vi "EOL Save Module Test Data v2.6.vi"(8 "error in":errorcluster, 11 "main state cluster":T1={"Application Status"="", "Switch Output Array"=[], "Switch Value Configuration"=[], "NVH Configuration"={"NVH Station?"=FALSE, "nvh app instance path"="", "NVH_ErrorMessages sv url"="", "NVH_Inputs sv url"="", "NVH_MotionNumber sv url"="", "NVH_Outputs sv url"="", "NVH_PartNumber sv url"="", "NVH_PartNumber_Echo sv url"="", "NVH_SerialNumber sv url"="", "NVH_AmbientTempF sv url"=""}, "rs232 port map"={"PMAC"="", "PS Port"="", "LVDT Unit"="", "RS232"=""}, "ethernet address map"={"LVDT 1 Unit"="172.17.53.143", "LVDT Unit 1 port"=0}, "paths"={"Base Path"=path "", "system error log path"=path "", "Error Table Path"=path "C/Labview Code/System/Error Table", "Store errors log path"=path "C/Labview Code/System/Error Table", "data bytes log path"=path "C/Labview Code/System/Error Table", "network path"=path "C/Labview Code/System/Error Table"}, "Station Index"=0, "Store Data"={"Motion Data Array"=[], "Error Table"=[], "Sun Shade Close Force Limits"={"Overall Min"=0.0, "Overall Max"=0.0, "Avg Min"=0.0, "Avg Max"=0.0, "Truncation Start"=0.0, "Truncation End"=0.0, "Variance"=0.0, "Check Noise"=FALSE}, "Sun Shade Open Force Limits"={"Overall Min"=0.0, "Overall Max"=0.0, "Avg Min"=0.0, "Avg Max"=0.0, "Truncation Start"=0.0, "Truncation End"=0.0, "Variance"=0.0, "Check Noise"=FALSE}, "Sunshade Open Data"=[], "Sunshade Close Data"=[], "Module Info"={"Serial Number"="", "Pallet Number"="", "Sunshade Color"="", "Inalfa Part Number"="", "Customer Number"=""}, "Sunsahde Close Raw Data"=[], "Sunshade Open Raw Data"=[], "Software Version"=[], "Constant Version"=[], "Hardware Version"=[], "Inalfa Part Number ECU"=[], "LVDT Data"=[], "Communication Line 1"=[], "Communication Line 2"=[], "Anti Pinch Force"=[], "Cycle Time"="", "Anti Pinch Vent Force"=[], "iGPS LVDT Data"=[], "data bytes log"=""}, "D in map"={"Abort Test"=enum."Dev2/port2/line6", "Start Test"=enum."Dev2/port2/line6"}, "DO Task"="", "ctl refs"={"Start Test"=refnum, "Abort Test"=refnum, "Manual Control"=refnum, "Route to Repair"=refnum, "Waveform Graph"=refnum, "Motion Data"=refnum, "all station status"=refnum, "Individual Station Status"=refnum, "exit program"=refnum, "Sunshade Servo Data Open"=refnum, "Sunshade Servo Data Close"=refnum, "Red-Rabbit Mode"=refnum, "Direct Manual Ctrl"=refnum}, "misc station config"={"Station Name"="", "is AT station?"=FALSE, "is audit station?"=FALSE, "power supply type"=enum."GENser", "use alt China TP2 LVDT Logic Seq"=FALSE, "hmi operator abort timeout"=0, "dump all analog values even if pass"=FALSE, "debug log pre-filter ap stream bytes"=FALSE, "use separate lvdt x and z extend tags"=FALSE, "is print"=FALSE}, "ethernet tcp refs"={"LVDT Unit"=refnum}, "Sunshade Barcode Scan"={"Sunshade Number 2"="", "Sunshade Number 1"="", "Keyence tuning bank idx"=0}, "AP Test Data"={"Raw Sunshade AP Data"="", "Raw Glass AP Data"="", "PMAC Read Counter"=0.0, "Database AP Data"=[]}, "Motion Status"={"hmi operator abort start time"=0, "Current Data Index"=0, "Analog Data"=[], "Motor Position Hex"=0, "Messages Index"=0, "Last Bytes"=[], "Current Hall Position"=0, "Motion Stop Timer"=0, "Position Test"=enum."Not Tested", "Noise Test"=enum."Not Tested", "motion stop check initialized"=FALSE, "remote sense enabled"=FALSE, "Motion"=enum."Glass Teach"}, "LVDT Status"={"LVDT's stored config"=[], "lvdt precision"={"truncate instead of rounding"=FALSE, "decimal places"=0}}, "Sequence State"={"Step Description"="", "Cycle Start Time"=0, "Step Data String"="", "Pass?"=FALSE, "Seqence"=[], "Active Step"=0, "Testing?"=FALSE, "Red-Rabbit Mode"=FALSE, "route-to-repair mode"=FALSE, "NVH Status"={"Restart IRQ Counter"=0, "NVH Test Needed?"=FALSE, "NVH Test Running?"=FALSE}, "Present (s)"=0.0, "Hold Mode?"=FALSE, "Hold?"=FALSE, "Rx Invalid?"=FALSE}, "misc status"={"delay start time (ticks)"=0, "In Vehicle Mode?"=FALSE, "Diag Mode?"=FALSE, "Serial Port Configured?"=FALSE, "PS Voltage"=0.0, "Diag Serial Port"="", "Part Setup"={"Communication Type"=enum."None", "Send Messages to"=enum."Glass", "RAP Signal"=enum."High", "Motor Type"=enum."Smart Motor", "NVH Part Number"=0, "Turn Off Timer"=0, "Part Type"=""}, "Part History Number"="", "Plant Number"=0, "AP Data Type"=enum."91/61", "Real Rollo?"=FALSE}, "NVH Operator?"=FALSE, "NVH Pass?"=FALSE, "Operator Pass?"=FALSE, "Operator Action?"=FALSE, "Noise Source"=0, "USBHandle"=0, "PeakInfo"="", "PeakNumber"=0, "NVH Motion Steps"=[], "Second Check?"=FALSE, "Decibel data"=[], "Direct Control Info"={"EnableStopOnHome"=FALSE, "EnableStopOnPos"=FALSE, "TeachEvent"=FALSE, "open offset"=0, "close offset"=0, "Derect control"=FALSE, "set position"=[], "teach pass "=FALSE, "Drift offsets"=[], "Hall Positions"=[]}, "manual control(direct)"=FALSE, "LIN INFO"={"Toolkit Type"=enum."Inalfa LIN", "NAD"=36, "Inalfa LIN"={"Master Frame(3C)"="", "Slave Frame(3D)"="NIXNET_exampleLDF", "Request Schedule"="NIXNET_exampleLDF", "Response Schedule"="CEMLIN3DiagResponseSchedule\nSPA3414_ConfigurationsCMAGeely_CEMCALYPSOSDB34XX0Cfg_LIN3_190709_", "Frame Write SCU"="", "Frame Read SCU"="", "LIN Name"=""}, "ADCS LIN"={"Port"="MasterReq\nSPA3414_ConfigurationsCMAGeely_CEMCALYPSOSDB34XX0Cfg_LIN3_190709_", "HW select"=0, "XNET Cluster"="SlaveResp\nSPA3414_ConfigurationsCMAGeely_CEMCALYPSOSDB34XX0Cfg_LIN3_190709_", "ByteCmd Path"=path "C/Labview Code/System/ByteCmdConfig.txt"}, "TS LIN"={"ref info"=refnum, "LIN Channel"=0, "ByteCmd Path"=path "C/Labview Code/System/ByteCmdConfig.txt"}}, "Config Info"=variant} {"LIN INFO"."NAD" format="%.0x"; "LIN INFO"."ADCS LIN"."HW select" items=["NI-XNET", "NI-CAN"]; "LVDT Status"."LVDT's stored config"."Lower Limit" format="%.2f"; "LVDT Status"."LVDT's stored config"."Upper Limit" format="%.2f"; "Store Data"."Sun Shade Open Force Limits"."Variance" format="%.2g"; "Store Data"."Sun Shade Open Force Limits"."Truncation End" format="%.2g"; "Store Data"."Sun Shade Open Force Limits"."Truncation Start" format="%.2g"; "Store Data"."Sun Shade Open Force Limits"."Avg Max" format="%.2g"; "Store Data"."Sun Shade Open Force Limits"."Avg Min" format="%.2g"; "Store Data"."Sun Shade Open Force Limits"."Overall Max" format="%.2g"; "Store Data"."Sun Shade Open Force Limits"."Overall Min" format="%.2g"; "Store Data"."Sun Shade Close Force Limits"."Variance" format="%.2g"; "Store Data"."Sun Shade Close Force Limits"."Truncation End" format="%.2g"; "Store Data"."Sun Shade Close Force Limits"."Truncation Start" format="%.2g"; "Store Data"."Sun Shade Close Force Limits"."Avg Max" format="%.2g"; "Store Data"."Sun Shade Close Force Limits"."Avg Min" format="%.2g"; "Store Data"."Sun Shade Close Force Limits"."Overall Max" format="%.2g"; "Store Data"."Sun Shade Close Force Limits"."Overall Min" format="%.2g"; "Store Data"."Motion Data Array"."Motion Data Limits"."LIN Msg"."Msg" format="%02x"; "Store Data"."Motion Data Array"."Motion Data Limits"."LIN Msg"."ID" format="%02x"}) -> (0 "error out":errorcluster)   [LabVIEW 2018]
uses:
  02.Type Def's/main state cluster.ctl
  02.Type Def's/All Switch Configuration Cluster.ctl
  02.Type Def's/All Motions.ctl
  02.Type Def's/EOL Switch Value Configuration Cluster.ctl
  02.Type Def's/EOL Switch Max Min Check Cluster.ctl
  02.Type Def's/station nvh config.ctl
  02.Type Def's/station rs232 port map.ctl
  02.Type Def's/station ethernet address map.ctl
  02.Type Def's/station paths.ctl
  02.Type Def's/EOL Save Module Test Data Control.ctl
  02.Type Def's/EOL Motion Database Table.ctl
  05.UserVI's/type defs/17x Audit Motion Data Seq Control.ctl
  05.UserVI's/type defs/17x AP Data Type.ctl
  05.UserVI's/type defs/17x Sunshade Limts Seq.ctl
  02.Type Def's/EOL Module Info Control.ctl
  02.Type Def's/station DI map.ctl
  05.UserVI's/type defs/EOL Global Digital Input Control.ctl
  02.Type Def's/control refs.ctl
  02.Type Def's/station motion data indicator.ctl
  02.Type Def's/Screen Motion Data.ctl
  02.Type Def's/Pass Fail Control.ctl
  02.Type Def's/station hmi.ctl
  02.Type Def's/lvdt name val pair.ctl
  02.Type Def's/individual station status.ctl
  02.Type Def's/misc station config.ctl
  05.UserVI's/Lambda Power/power supply types.ctl
  05.UserVI's/type defs/EOL LVDT's Check Controller.ctl
  05.UserVI's/LVDT's/lvdt precision.ctl
  02.Type Def's/sequence state.ctl
  05.UserVI's/sequence/type defs/Sequence Info.ctl
  05.UserVI's/type defs/EOL Part Setup.ctl
  02.Type Def's/All Communication Types.ctl
  05.UserVI's/type defs/Communication with Motors.ctl
  05.UserVI's/type defs/RAP Signal Control.ctl
  05.UserVI's/type defs/EOL Motor Type.ctl
  02.Type Def's/station LIN config.ctl
  03.Inalfa LIN/LIN Device.ctl
  <vilib>/CMC.AME/Inalfa ADCS/Ctl'Def/ADCS_LIN info.ctl
  C:/Program Files (x86)/National Instruments/LabVIEW 2018/vi.lib/CMC.AME/Inalfa TS LIN/TOSUN/TSMaster/bin/Interop.TSMasterAPI.dll
  Program Files (x86)/National Instruments/LabVIEW 2018/vi.lib/CMC.AME/Inalfa TS LIN/TOSUN/TSMaster/bin/Interop.TSMasterAPI.dll
  06.Test Loop/Sub'VIs/Type Def's/Config Info.ctl
  <vilib>/Utility/file.llb/Write To Spreadsheet File (string).vi
panel:
  in  "Store Sunshade Raw Data?":bool
  # "Sunroof Barcode"
  # "Pallet Number"
  # "Part Type"
  # "Application Status"
  # "Current Step"
  # "Cycle Time"
  # "Pass / Fail"
  # "Shade Close"
  # "Actual Data"
  # "Limits"
  # "Avg Current"
  # "Run Time"
  # "Speed"
  # "Noise Test"
  # "Position"
  # "Shade Open"
  # "Actual Data"
  # "Limits"
  # "Avg Current"
  # "Run Time"
  # "Speed"
  # "Noise Test"
  # "Position"
  # "Vent Close"
  # "Actual Data"
  # "Limits"
  # "Avg Current"
  # "Run Time"
  # "Speed"
  # "Noise Test"
  # "Position"
  # "Vent Open"
  # "Actual Data"
  # "Limits"
  # "Avg Current"
  # "Run Time"
  # "Speed"
  # "Noise Test"
  # "Position"
  # "Slide Close"
  # "Actual Data"
  # "Limits"
  # "Avg Current"
  # "Run Time"
  # "Speed"
  # "Noise Test"
  # "Position"
  # "Slide Open"
  # "Actual Data"
  # "Limits"
  # "Avg Current"
  # "Run Time"
  # "Speed"
  # "Noise Test"
  # "Position"
  # "Min"
  # "N"
  # "Min"
  # "Start"
  # "N"
  # "Max"
  # "N"
  # "Max"
  # "N"
  # "End"
  # "Min"
  # "N"
  # "Min"
  # "Start"
  # "N"
  # "Max"
  # "N"
  # "Max"
  # "N"
  # "End"
  # "Min"
  # "Max"
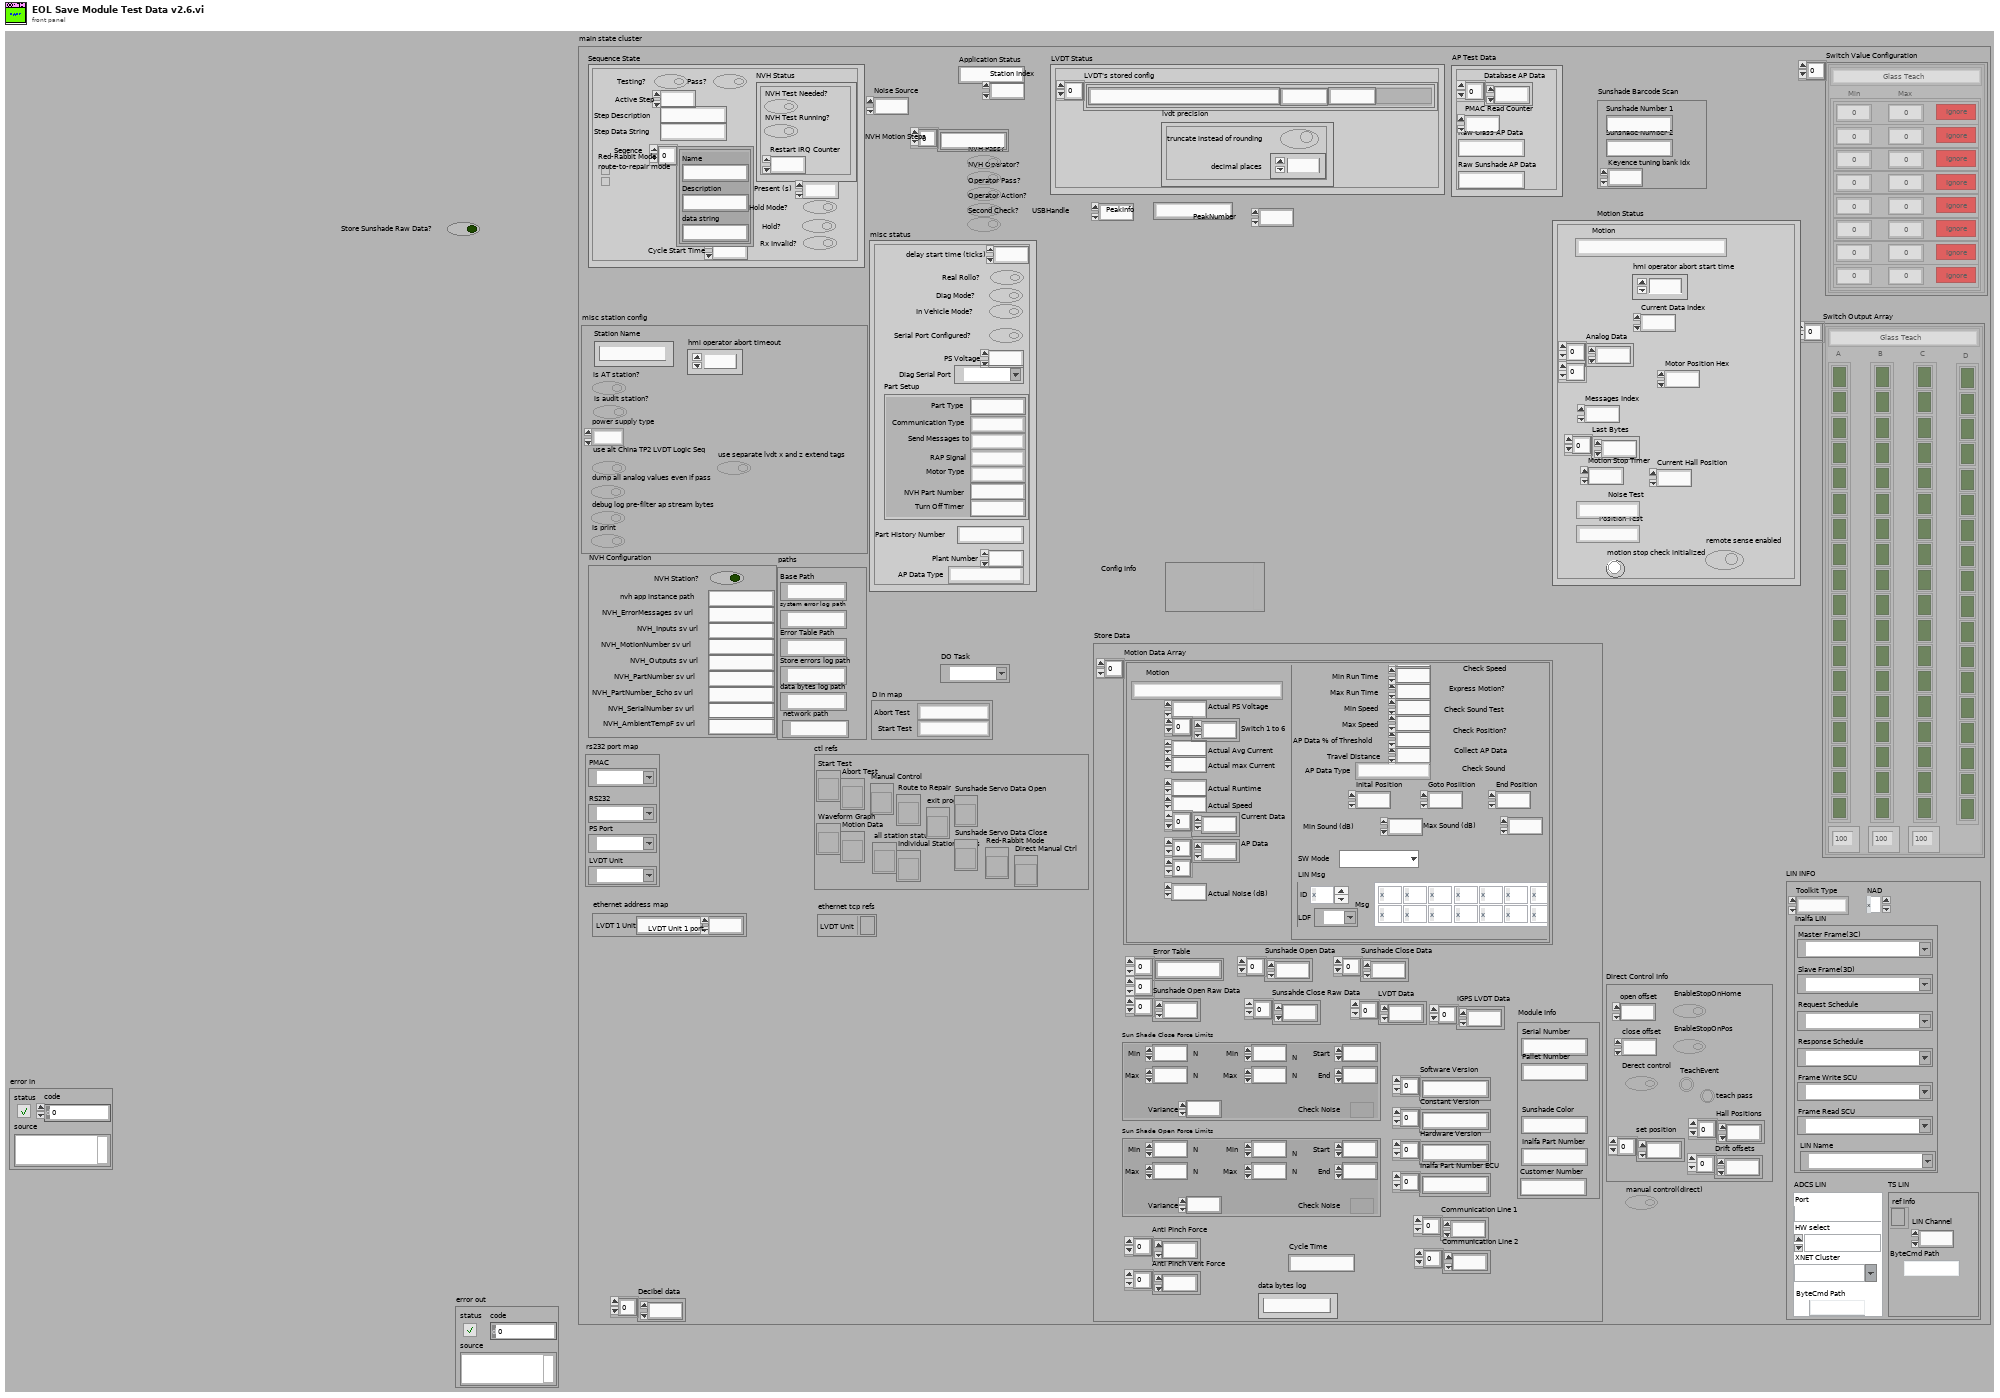
[diagram p1: front panel]
types:
  T1 = typedef "main state cluster.ctl" = cluster{"Application Status":string, "Switch Output Array":T2[], "Switch Value Configuration":T4[], "NVH Configuration":T6, "rs232 port map":T7, "ethernet address map":T8, "paths":T9, "Station Index":i32, "Store Data":T10, "D in map":T16, "DO Task":refnum<k21>, "ctl refs":T18, "misc station config":T19, "ethernet tcp refs":cluster{"LVDT Unit":refnum<k5>}, "Sunshade Barcode Scan":cluster{"Sunshade Number 2":string, "Sunshade Number 1":string, "Keyence tuning bank idx":i32}, "AP Test Data":cluster{"Raw Sunshade AP Data":string, "Raw Glass AP Data":string, "PMAC Read Counter":dbl, "Database AP Data":dbl[]}, "Motion Status":cluster{"hmi operator abort start time":u32, "Current Data Index":i32, "Analog Data":sgl[][], "Motor Position Hex":u16, "Messages Index":u16, "Last Bytes":u8[], "Current Hall Position":i16, "Motion Stop Timer":u32, "Position Test":T21, "Noise Test":T21, "motion stop check initialized":bool, "remote sense enabled":bool, "Motion":T3}, "LVDT Status":cluster{"LVDT's stored config":T22[], "lvdt precision":T23}, "Sequence State":T24, "misc status":cluster{"delay start time (ticks)":u32, "In Vehicle Mode?":bool, "Diag Mode?":bool, "Serial Port Configured?":bool, "PS Voltage":dbl, "Diag Serial Port":refnum<visa-resource-name>, "Part Setup":T26, "Part History Number":string, "Plant Number":u8, "AP Data Type":T13, "Real Rollo?":bool}, "NVH Operator?":bool, "NVH Pass?":bool, "Operator Pass?":bool, "Operator Action?":bool, "Noise Source":u32, "USBHandle":i32, "PeakInfo":string, "PeakNumber":i32, "NVH Motion Steps":string[], "Second Check?":bool, "Decibel data":dbl[], "Direct Control Info":cluster{"EnableStopOnHome":bool, "EnableStopOnPos":bool, "TeachEvent":bool, "open offset":i32, "close offset":i32, "Derect control":bool, "set position":i32[], "teach pass ":bool, "Drift offsets":i32[], "Hall Positions":i32[]}, "manual control(direct)":bool, "LIN INFO":T31, "Config Info":T34}
  T2 = typedef "All Switch Configuration Cluster.ctl" = cluster{"All Motions":T3, "A":bool[], "B":bool[], "C":bool[], "D":bool[], "A activation time (ms)":u32, "B activation time (ms)":u32, "C activation time (ms)":u32}
  T3 = typedef "All Motions.ctl" = enum16{"Glass Teach", "Glass Slide Open", "Glass Slide Close", "Glass Vent Open", "Glass Vent Close", "Sunshade Teach", "Sunshade Open", "Sunshade Close", "Idle", "Sunshade Open 2", "Sunshade Close 2", "Glass Slide Open Sunshade Open", "Glass Slide Open Sunshade Close", "Glass Slide Close Sunshade Open", "Glass Slide Close Sunshade Close", "Glass Vent Open Sunshade Open", "Glass Vent Open Sunshade Close", "Glass Vent Close Sunshade Open", "Glass Vent Close Sunshade Close", "Express Glass Slide Open", "Express Glass Slide Close", "Express Glass Vent Open", "Express Glass Vent Close", "Express Sunshade Open", "Express Sunshade Close", "Express Sunshade Open 2", "Express Sunshade Close 2", "Express Glass Slide Open Sunshade Open", "Express Glass Slide Open Sunshade Close", "Express Glass Slide Close Sunshade Open", "Express Glass Slide Close Sunshade Close", "Express Glass Vent Open Sunshade Open", "Express Glass Vent Open Sunshade Close", "Express Glass Vent Close Sunshade Open", "Express Glass Vent Close Sunshade Close", "Goto Position Glass", "Goto Position Sunshade", "Sunshade Teach 2"}
  T4 = typedef "EOL Switch Value Configuration Cluster.ctl" = cluster{"All Motions":T3, "Array":T5[]}
  T5 = typedef "EOL Switch Max Min Check Cluster.ctl" = cluster{"Min":dbl, "Max":dbl, "Check?":bool}
  T6 = typedef "station nvh config.ctl" = cluster{"NVH Station?":bool, "nvh app instance path":string, "NVH_ErrorMessages sv url":string, "NVH_Inputs sv url":string, "NVH_MotionNumber sv url":string, "NVH_Outputs sv url":string, "NVH_PartNumber sv url":string, "NVH_PartNumber_Echo sv url":string, "NVH_SerialNumber sv url":string, "NVH_AmbientTempF sv url":string}
  T7 = typedef "station rs232 port map.ctl" = cluster{"PMAC":refnum<visa-resource-name>, "PS Port":refnum<visa-resource-name>, "LVDT Unit":refnum<visa-resource-name>, "RS232":refnum<visa-resource-name>}
  T8 = typedef "station ethernet address map.ctl" = cluster{"LVDT 1 Unit":string, "LVDT Unit 1 port":u16}
  T9 = typedef "station paths.ctl" = cluster{"Base Path":path, "system error log path":path, "Error Table Path":path, "Store errors log path":path, "data bytes log path":path, "network path":path}
  T10 = typedef "EOL Save Module Test Data Control.ctl" = cluster{"Motion Data Array":T11[], "Error Table":string[][], "Sun Shade Close Force Limits":T14, "Sun Shade Open Force Limits":T14, "Sunshade Open Data":sgl[], "Sunshade Close Data":sgl[], "Module Info":T15, "Sunsahde Close Raw Data":sgl[], "Sunshade Open Raw Data":sgl[], "Software Version":string[], "Constant Version":string[], "Hardware Version":string[], "Inalfa Part Number ECU":string[], "LVDT Data":sgl[], "Communication Line 1":sgl[], "Communication Line 2":sgl[], "Anti Pinch Force":sgl[], "Cycle Time":string, "Anti Pinch Vent Force":sgl[], "iGPS LVDT Data":sgl[], "data bytes log":string}
  T11 = typedef "EOL Motion Database Table.ctl" = cluster{"Motion":T3, "Actual Avg Current":dbl, "Actual Runtime":dbl, "Actual Speed":dbl, "Current Data":sgl[], "Motion Data Limits":T12, "Switch 1 to 6":dbl[], "Actual PS Voltage":dbl, "AP Data":i16[][], "Actual max Current":dbl, "Actual Noise (dB)":dbl}
  T12 = typedef "17x Audit Motion Data Seq Control.ctl" = cluster{"Power Supply Voltage":dbl, "Min Avg Current":dbl, "Max Avg Current":dbl, "Min Run Time":dbl, "Max Run Time":dbl, "Min Speed":dbl, "Max Speed":dbl, "AP Data % of Threshold":dbl, "Travel Distance":dbl, "AP Data Type":T13, "Check Current":bool, "Check Run Time":bool, "Check Speed":bool, "Express Motion?":bool, "Check Sound Test":bool, "Check Position?":bool, "Collect AP Data":bool, "Inital Position":u16, "End Position":u16, "Goto Posiition":u16, "Max max Current":dbl, "Min max Current":dbl, "Check max Current":bool, "Check Sound":bool, "Min Sound (dB)":dbl, "Max Sound (dB)":dbl, "SW Mode":enum16{"Hard Switch", "Uncond Frame"}, "LIN Msg":cluster{"ID":u8, "Msg":u8[][], "LDF":refnum<k21>}}
  T13 = typedef "17x AP Data Type.ctl" = enum16{"91/61", "92/62", "93/63", "67", "68", "6F", "71", "91 Msg", "92 Msg", "93 Msg", "94 Msg", "HiRain 91", "HiRain 92 Speed", "HiRain 92 HS", "HiRain 92", "HiRain 93", "SnT"}
  T14 = typedef "17x Sunshade Limts Seq.ctl" = cluster{"Overall Min":dbl, "Overall Max":dbl, "Avg Min":dbl, "Avg Max":dbl, "Truncation Start":dbl, "Truncation End":dbl, "Variance":dbl, "Check Noise":bool}
  T15 = typedef "EOL Module Info Control.ctl" = cluster{"Serial Number":string, "Pallet Number":string, "Sunshade Color":string, "Inalfa Part Number":string, "Customer Number":string}
  T16 = typedef "station DI map.ctl" = cluster{"Abort Test":T17, "Start Test":T17}
  T17 = typedef "EOL Global Digital Input Control.ctl" = enum16{"Dev2/port0/line0", "Dev2/port0/line1", "Dev2/port0/line2", "Dev2/port0/line3", "Dev2/port0/line4", "Dev2/port0/line5", "Dev2/port0/line6", "Dev2/port0/line7", "Dev2/port1/line0", "Dev2/port1/line1", "Dev2/port1/line2", "Dev2/port1/line3", "Dev2/port1/line4", "Dev2/port1/line5", "Dev2/port1/line6", "Dev2/port1/line7", "Dev2/port2/line0", "Dev2/port2/line1", "Dev2/port2/line2", "Dev2/port2/line3", "Dev2/port2/line4", "Dev2/port2/line5", "Dev2/port2/line6", "Dev2/port2/line7", "Prerun Start Test", "Prerun Abort Test", "Audit Start Test", "Audit Abort Test", "Dev2/port3/line4", "Dev2/port3/line5", "Breakin Start Test", "Breakin Abort Test", "Not Implemented"}
  T18 = typedef "control refs.ctl" = cluster{"Start Test":refnum<vi>, "Abort Test":refnum<vi>, "Manual Control":refnum<vi>, "Route to Repair":refnum<vi>, "Waveform Graph":refnum<vi>, "Motion Data":refnum<vi>, "all station status":refnum<vi>, "Individual Station Status":refnum<vi>, "exit program":refnum<vi>, "Sunshade Servo Data Open":refnum<vi>, "Sunshade Servo Data Close":refnum<vi>, "Red-Rabbit Mode":refnum<vi>, "Direct Manual Ctrl":refnum<vi>}
  T19 = typedef "misc station config.ctl" = cluster{"Station Name":string, "is AT station?":bool, "is audit station?":bool, "power supply type":T20, "use alt China TP2 LVDT Logic Seq":bool, "hmi operator abort timeout":u32, "dump all analog values even if pass":bool, "debug log pre-filter ap stream bytes":bool, "use separate lvdt x and z extend tags":bool, "is print":bool}
  T20 = typedef "power supply types.ctl" = enum16{"GENser", "ZUPser", "GENeth", "Manual", "ITECH"}
  T21 = typedef "Pass Fail Control.ctl" = enum16{"Not Tested", "Pass", "Fail"}
  T22 = typedef "EOL LVDT's Check Controller.ctl" = cluster{"Upper Limit":dbl, "Lower Limit":dbl, "LVDT Name":string, "Check":bool}
  T23 = typedef "lvdt precision.ctl" = cluster{"truncate instead of rounding":bool, "decimal places":u8}
  T24 = typedef "sequence state.ctl" = cluster{"Step Description":string, "Cycle Start Time":u32, "Step Data String":string, "Pass?":bool, "Seqence":T25[], "Active Step":u8, "Testing?":bool, "Red-Rabbit Mode":bool, "route-to-repair mode":bool, "NVH Status":cluster{"Restart IRQ Counter":u8, "NVH Test Needed?":bool, "NVH Test Running?":bool}, "Present (s)":dbl, "Hold Mode?":bool, "Hold?":bool, "Rx Invalid?":bool}
  T25 = typedef "Sequence Info.ctl" = cluster{"Name":string, "Description":string, "data string":string}
  T26 = typedef "EOL Part Setup.ctl" = cluster{"Communication Type":T27, "Send Messages to":T28, "RAP Signal":T29, "Motor Type":T30, "NVH Part Number":u16, "Turn Off Timer":u16, "Part Type":string}
  T27 = typedef "All Communication Types.ctl" = enum16{"None", "CAN", "RS 232", "RS 232 LIN", "GM LIN", "SnT LIN", "K Line", "Robel CAN", "P42M-Continental", "Inalfa SCU LIN", "Spare 3"}
  T28 = typedef "Communication with Motors.ctl" = enum16{"Glass", "Rollo", "Both"}
  T29 = typedef "RAP Signal Control.ctl" = enum16{"High", "Low", "None"}
  T30 = typedef "EOL Motor Type.ctl" = enum16{"Smart Motor", "Sensor Motor"}
  T31 = typedef "station LIN config.ctl" = cluster{"Toolkit Type":enum16{"Inalfa LIN", "ADCS LIN", "TS LIN"}, "NAD":u8, "Inalfa LIN":T32, "ADCS LIN":T33, "TS LIN":cluster{"ref info":refnum<k24>, "LIN Channel":i32, "ByteCmd Path":path}}
  T32 = typedef "LIN Device.ctl" = cluster{"Master Frame(3C)":refnum<k21>, "Slave Frame(3D)":refnum<k21>, "Request Schedule":refnum<k21>, "Response Schedule":refnum<k21>, "Frame Write SCU":refnum<k21>, "Frame Read SCU":refnum<k21>, "LIN Name":refnum<k21>}
  T33 = typedef "ADCS_LIN info.ctl" = cluster{"Port":string, "HW select":u16, "XNET Cluster":string, "ByteCmd Path":path}
  T34 = typedef "Config Info.ctl" = variant
  T35 = cluster{"Base Path":path, "Relative Path Excel Data":string, "Relative Path AP Data":string, "Relative Path Current Data":string, "Relative Path Sunshade Force Data":string, "Excel Data Array":string[], "Date n Time":string, "AP Data":i16[][][], "Current Data":sgl[][], "Relative Path Data Bytes Log":string, "Relative Path Analog Data":string, "main state cluster":T1, "Red Rabbit Relative Path Excel Data":string, "Route to repair relative path excel data":string, "bmw hall log relative path":string}
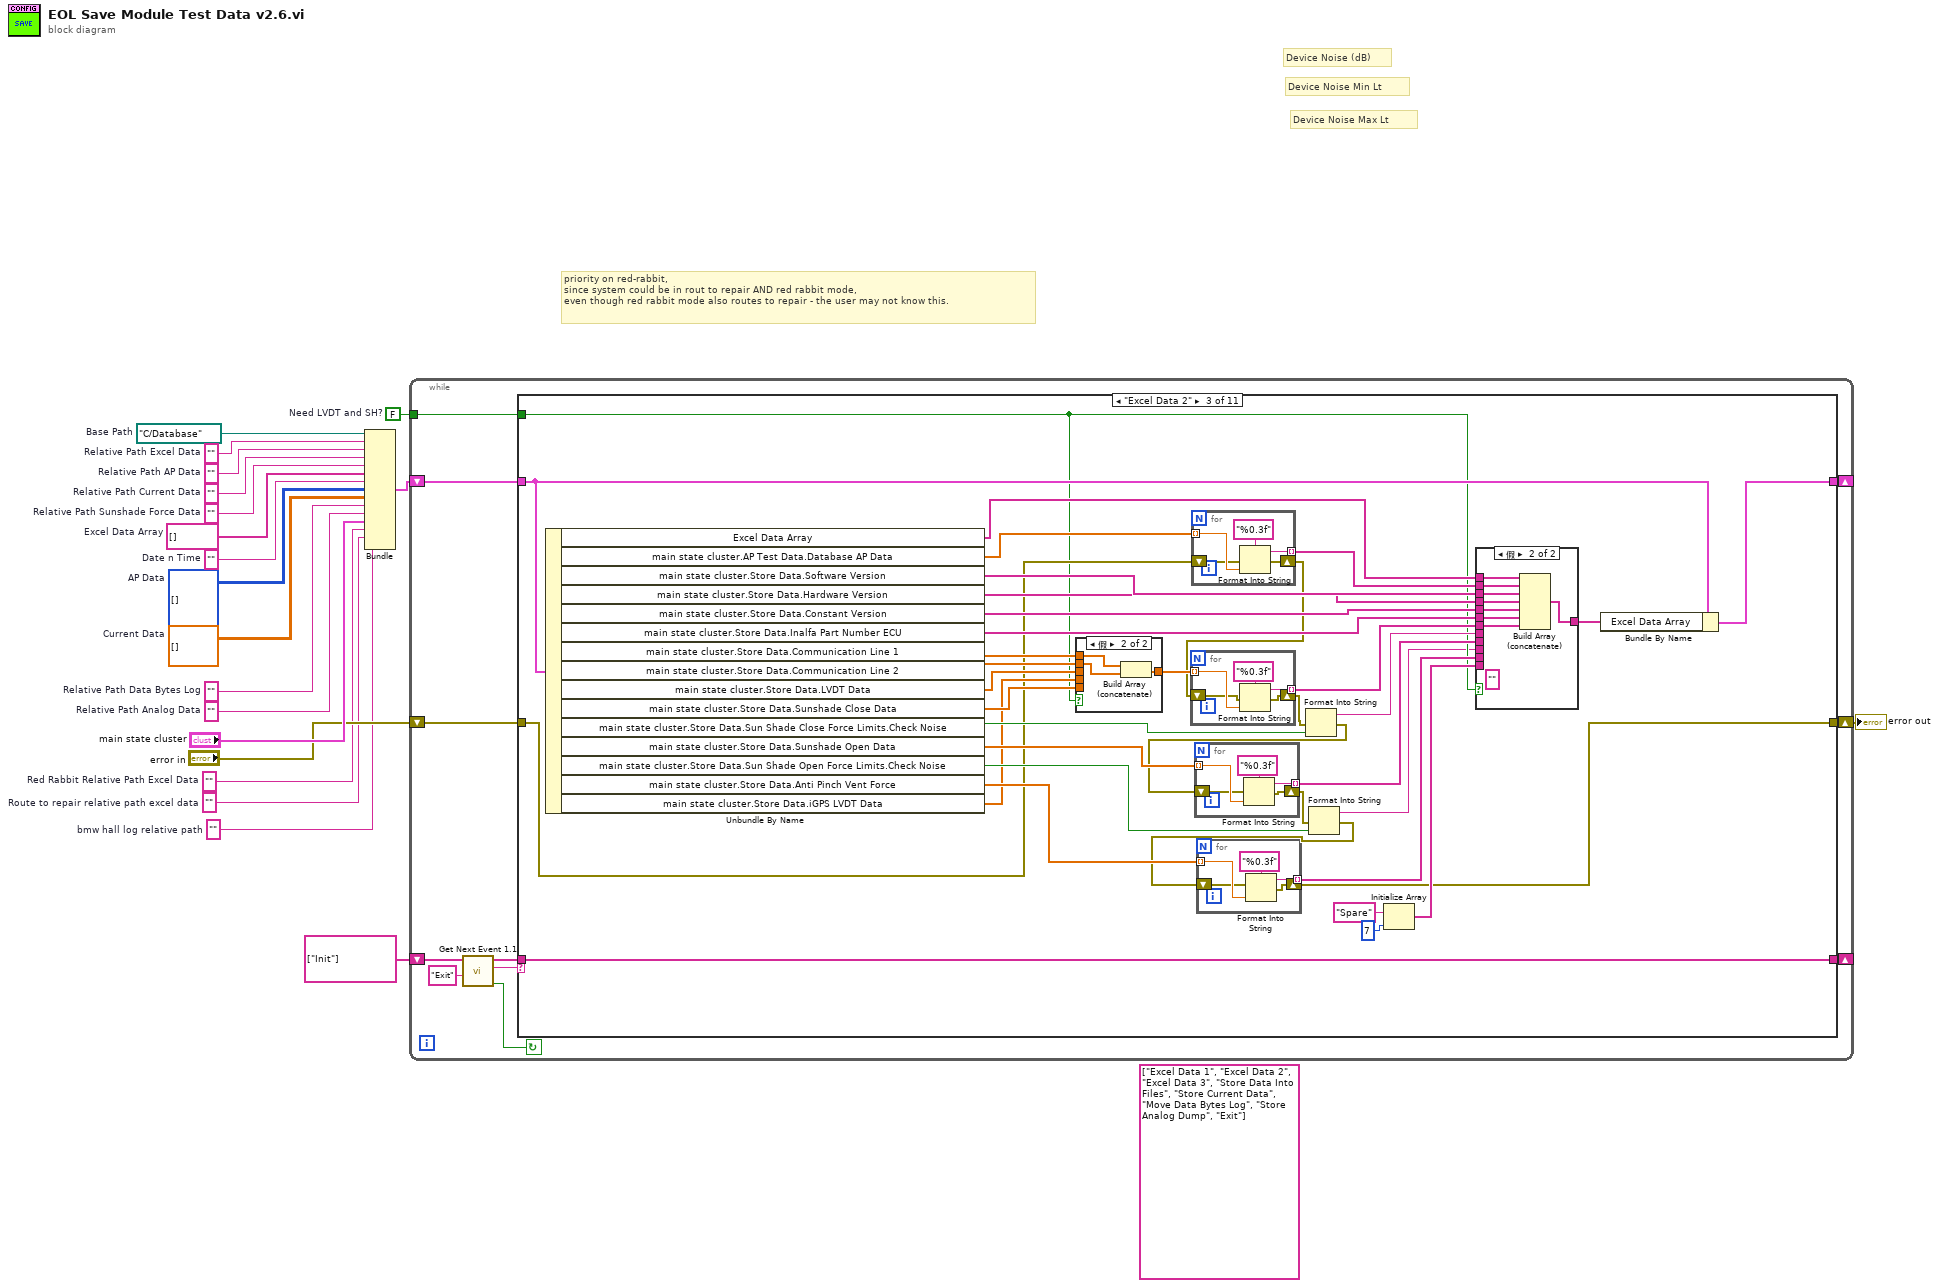
[diagram p0: block diagram]
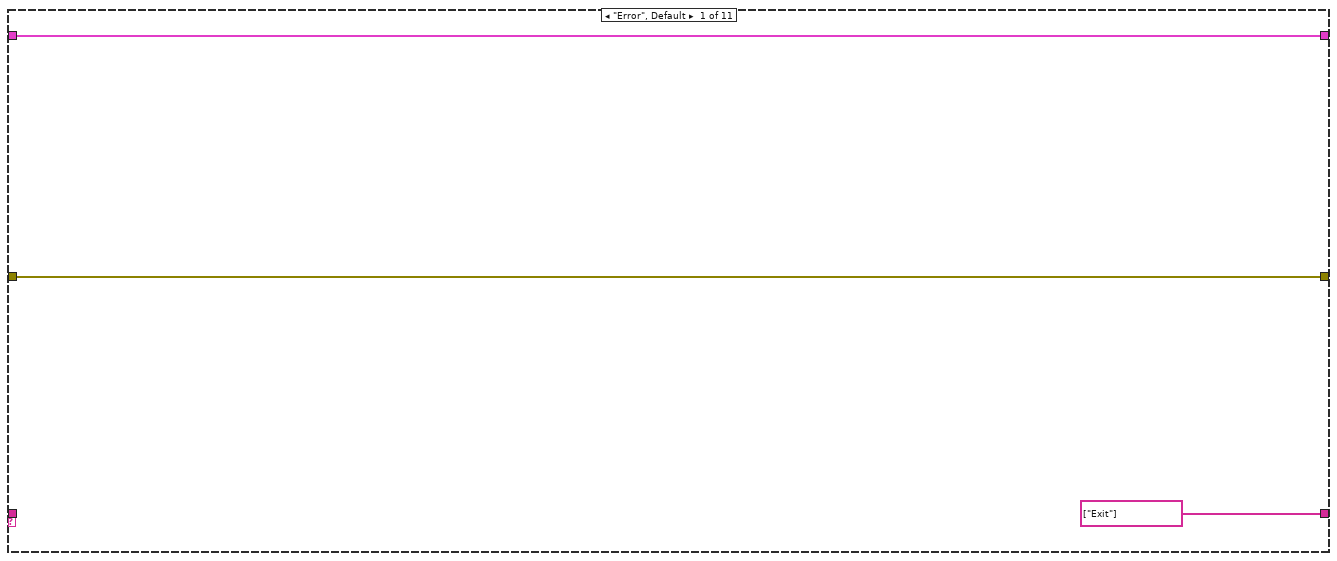
[diagram p2: hidden frame]
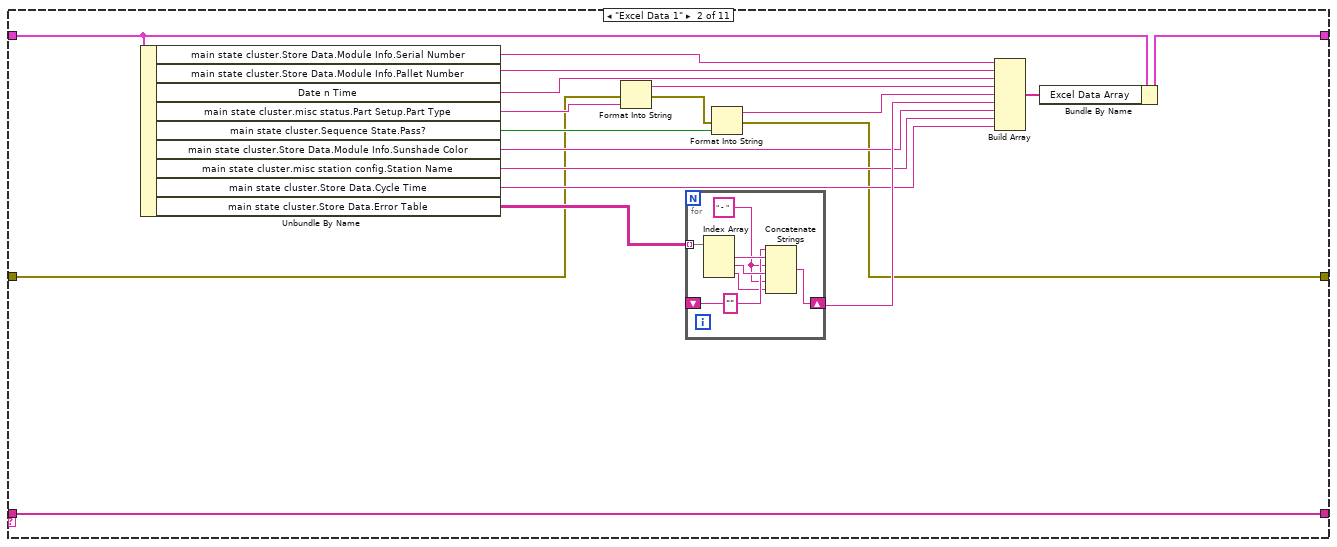
[diagram p3: hidden frame]
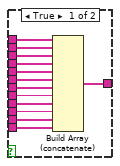
[diagram p4: hidden frame]
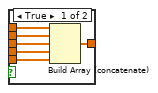
[diagram p5: hidden frame]
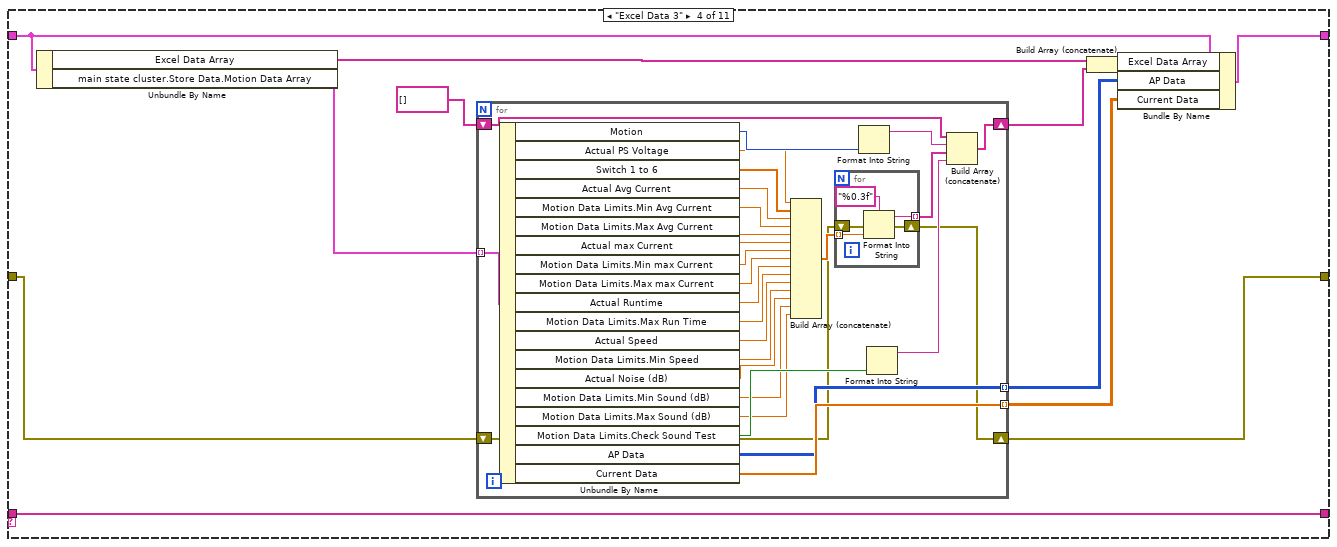
[diagram p6: hidden frame]
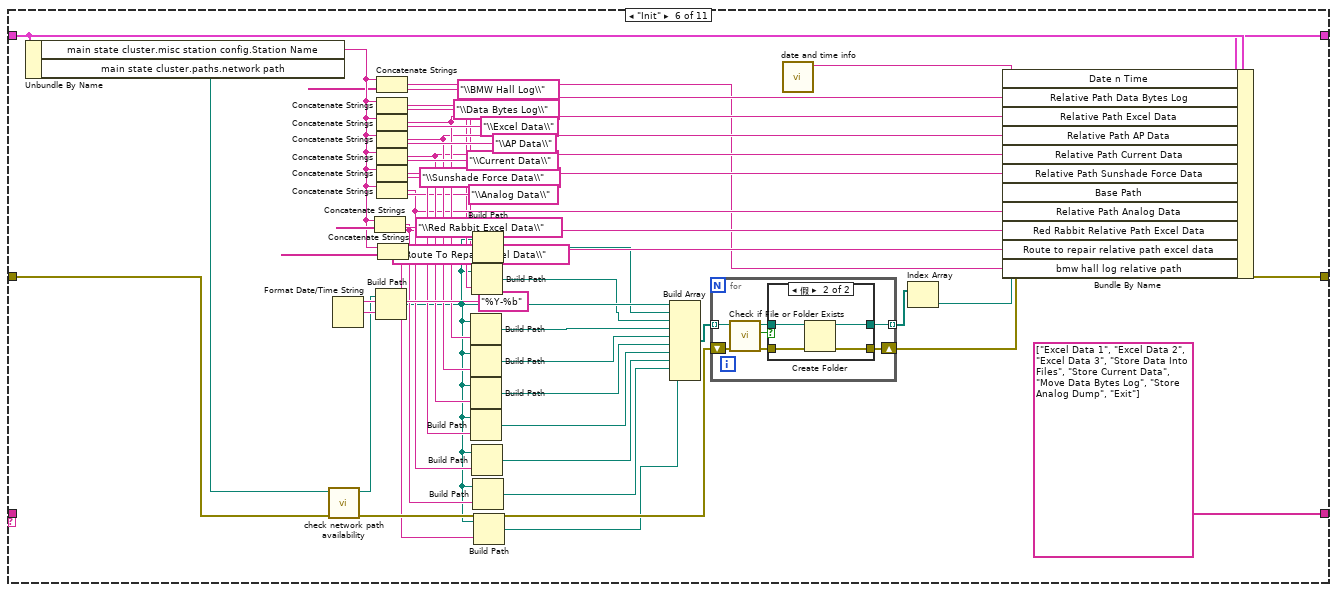
[diagram p8: hidden frame]
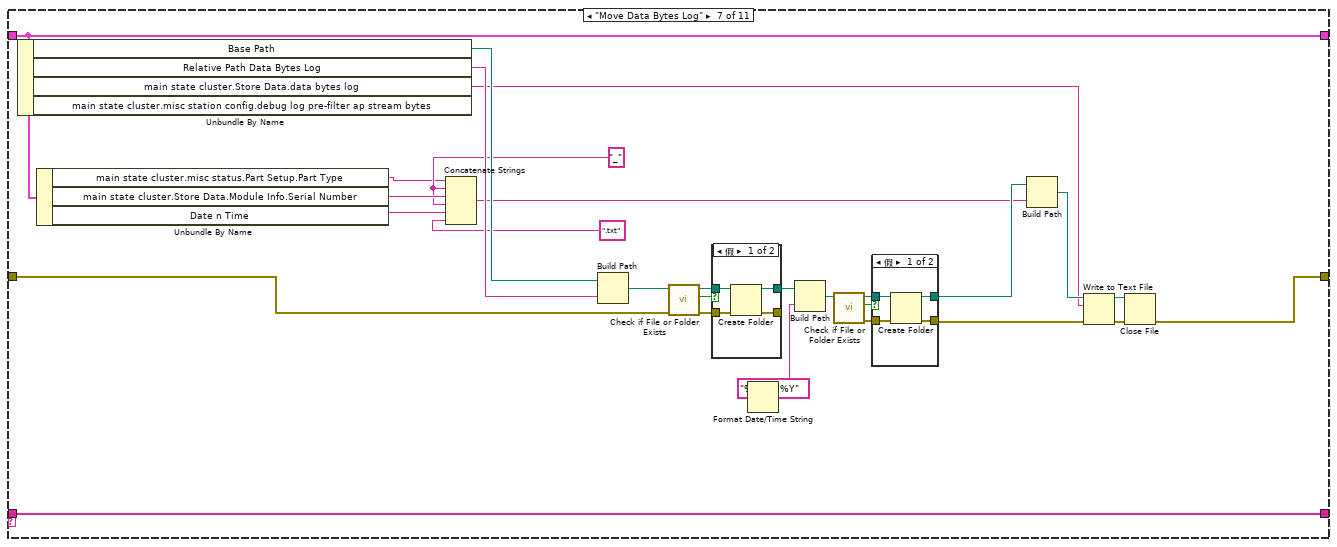
[diagram p10: hidden frame]
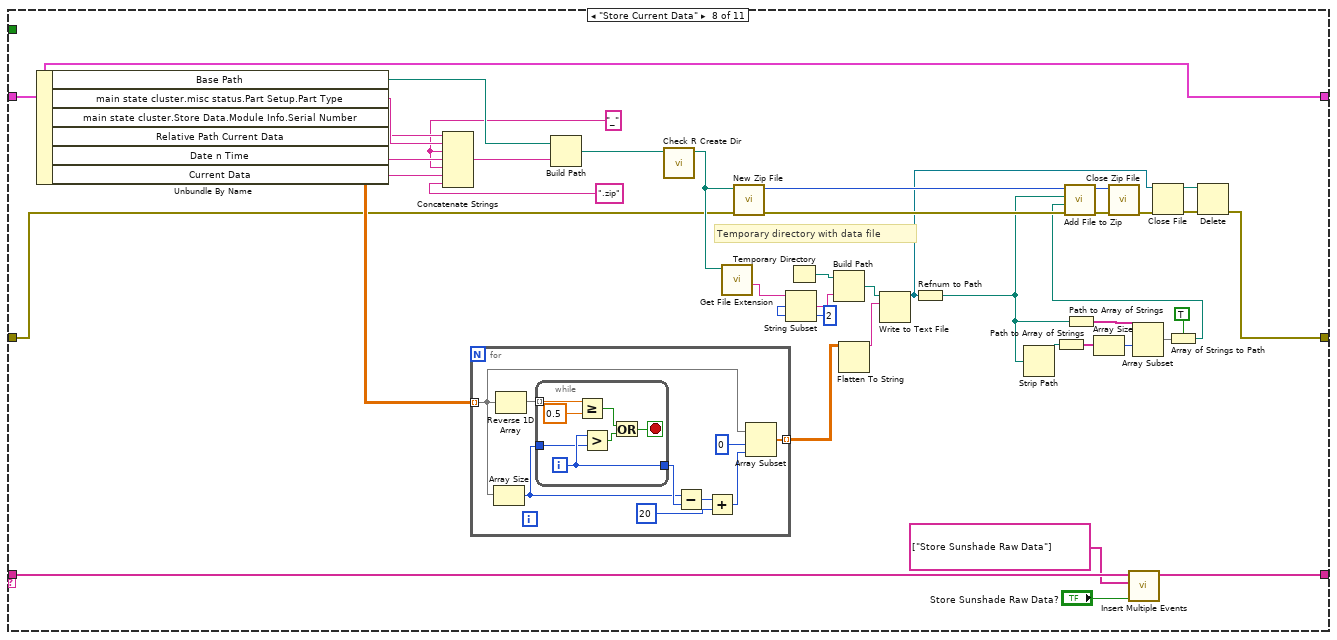
[diagram p13: hidden frame]
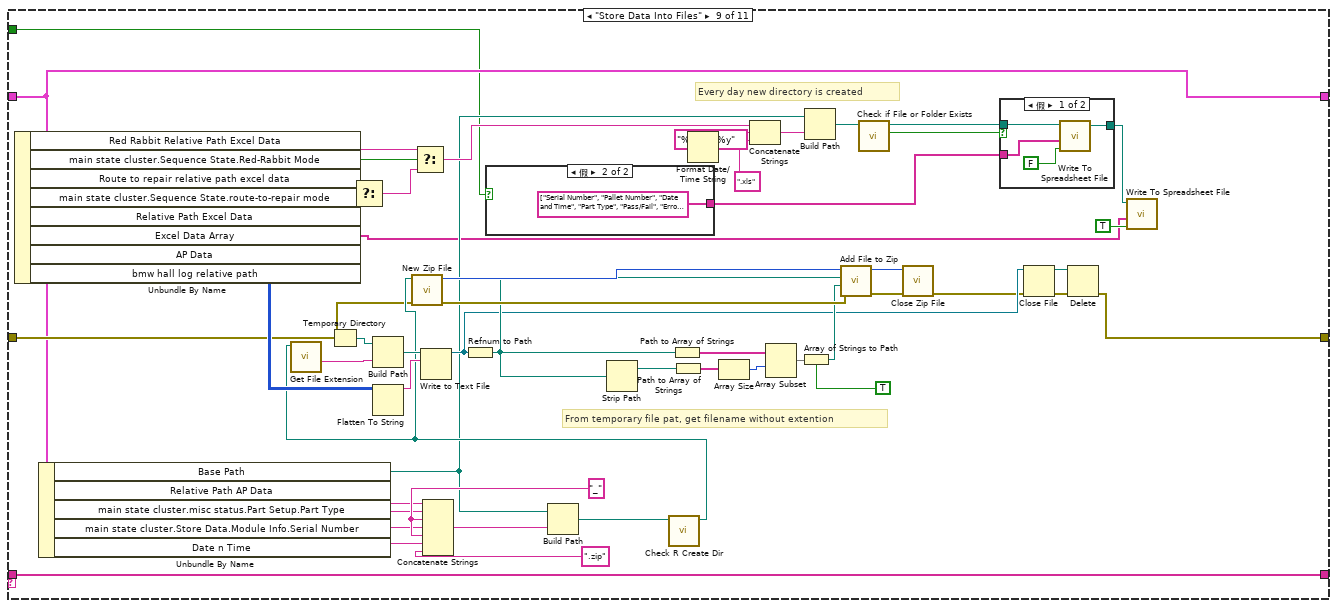
[diagram p14: hidden frame]
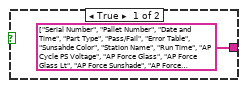
[diagram p15: hidden frame]
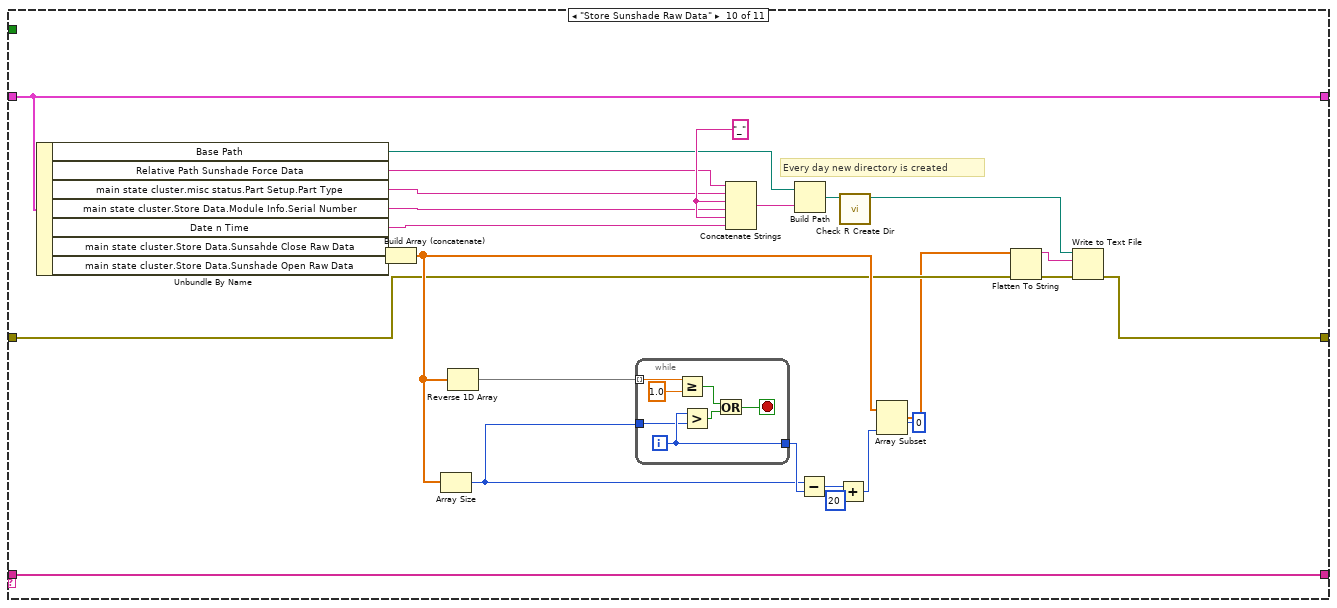
[diagram p17: hidden frame]
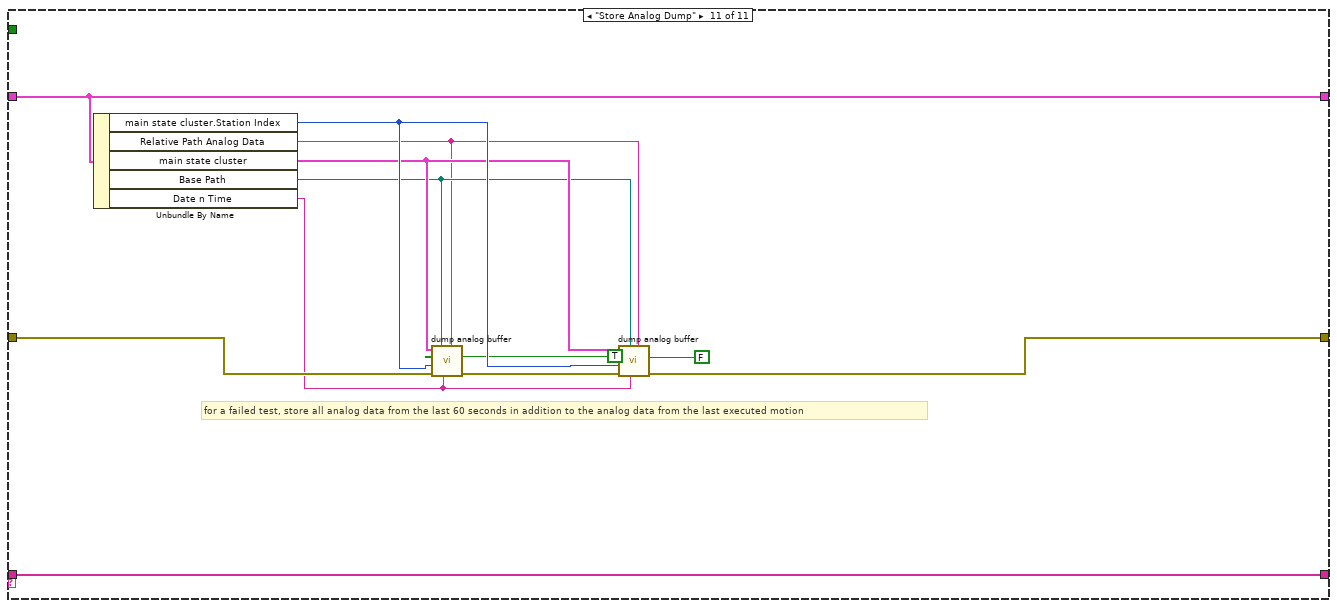
[diagram p18: hidden frame]
diagram:
  w1 = FALSE  # Need LVDT and SH?
  (unwired) string[] ["Excel Data 1", "Excel Data 2", "Excel Data 3", "Store Data Into Files", "Store Current Data", "Move Data Bytes Log", "Store Analog Dump", "Exit"] ("event queue out")
  w2 = ""  # bmw hall log relative path
  w3 = ""  # Route to repair relative path excel data
  w4 = ""  # Red Rabbit Relative Path Excel Data
  w8 = ""  # Relative Path Analog Data
  w9 = ""  # Relative Path Data Bytes Log
  w19 = path "C:/Database"  # Base Path
  w10 = sgl[][] []  # Current Data
  w11 = i16[][][] []  # AP Data
  w12 = ""  # Date n Time
  w13 = string[] []  # Excel Data Array
  w14 = ""  # Relative Path Sunshade Force Data
  w15 = ""  # Relative Path Current Data
  w16 = ""  # Relative Path AP Data
  w17 = ""  # Relative Path Excel Data
  # "priority on red-rabbit,\nsince system could be in rout to repair AND red rabbit mode,\neven though red rabbit mode also routes to repair - the user may not know this."
  # "Device Noise Max Lt"
  # "Device Noise Min Lt"
  # "Device Noise (dB)"
  n1 = Bundle("Base Path"=w19, "Relative Path Excel Data"=w17, "Relative Path AP Data"=w16, "Relative Path Current Data"=w15, "Relative Path Sunshade Force Data"=w14, "Excel Data Array"=w13, "Date n Time"=w12, "AP Data"=w11, "Current Data"=w10, "Relative Path Data Bytes Log"=w9, "Relative Path Analog Data"=w8, "main state cluster"="main state cluster", "Red Rabbit Relative Path Excel Data"=w4, "Route to repair relative path excel data"=w3, "bmw hall log relative path"=w2) -> (w18:T35)  [unwired: 1 in]
  n2 = while {
    shift-right: [w28] -> _
    shift-left: string[] ["Init"] ("event queue out") -> [w27]
    shift-right: [w25] -> _
    shift-left: w18 -> [w26]
    shift-right: [w22] -> w5
    shift-left: "error in" -> [w23]
    tunnel: w1 -> [w21]
    stop <- w31 continue-if-true
    n3 = call "Get Next Event 1.1.vi"("Exit Event"="Exit", "event queue in"=w27) -> ("Condition (Exit:F)"=w31:bool, "next event"=w30:string, "event queue out"=w29:string[])  [unwired: 6 in, 1 out]
    n4 = case shown="\"Excel Data 2\"" w30 {
      tunnel: w29 -> [_ w54 w98 w160 w195 _ w275 w333 w390 w437 w453]
      tunnel: [string[] ["Exit"] ("event queue out") w54 w98 w160 w195 string[] ["Excel Data 1", "Excel Data 2", "Excel Data 3", "Store Data Into Files", "Store Current Data", "Move Data Bytes Log", "Store Analog Dump", "Exit"] ("event queue out") w275 w332 w390 w437 w453] -> w28
      tunnel: w26 -> [w34 w51 w96 w159 w196 w239 w261 w296 w354 w413 w454]
      tunnel: [w34 w50 w95 w158 w196 w238 w261 w296 w354 w413 w454] -> w25
      tunnel: w23 -> [w32 w37 w70 w150 w194 w213 w266 w294 w364 w415 w452]
      tunnel: [w32 w35 w64 w149 w194 w212 w253 w295 w352 w414 w451] -> w22
      tunnel: w21 -> [_ _ w63 _ _ _ _ _ w351 _ _]
      frame "Error", Default {
      }
      frame "Excel Data 1" {
        n5 = Unbundle By Name(w51) -> ("main state cluster.Store Data.Module Info.Serial Number"=w53:string, "main state cluster.Store Data.Module Info.Pallet Number"=w52:string, "Date n Time"=w40:string, "main state cluster.misc status.Part Setup.Part Type"=w46:string, "main state cluster.Sequence State.Pass?"=w48:bool, "main state cluster.Store Data.Module Info.Sunshade Color"=w42:string, "main state cluster.misc station config.Station Name"=w38:string, "main state cluster.Store Data.Cycle Time"=w39:string, "main state cluster.Store Data.Error Table"=w41:string[][])
        n6 = Format Into String(error in=w37, w46) -> (resulting string=w45:string, error out=w36:errorcluster)  [unwired: 2 in]
        n7 = for {
          tunnel: w41 -> [w61] mode=indexing
          shift-right: [w58] -> w43
          shift-left: "" -> [w57]
          w56 = " - " ("string")
          n8 = Index Array(array=w61) -> (element #1=w60:string, element #2=w59:string, element #3=w55:string)  [unwired: 3 in]
          n9 = Concatenate Strings(w57, w60, w56, w59, w56, w55) -> (w58:string)
        }
        n10 = Format Into String(error in=w36, w48) -> (resulting string=w47:string, error out=w35:errorcluster)  [unwired: 2 in]
        n11 = Build Array(w53, w52, w40, w45, w47, w43, w42, w38, w39) -> (w49:string[])
        n12 = Bundle By Name(cluster=w51, "Excel Data Array"=w49) -> (w50:T35)
      }
      frame "Excel Data 2" {
        n13 = Unbundle By Name(w96) -> ("Excel Data Array"=w80:string[], "main state cluster.AP Test Data.Database AP Data"=w93:dbl[], "main state cluster.Store Data.Software Version"=w97:string[], "main state cluster.Store Data.Hardware Version"=w91:string[], "main state cluster.Store Data.Constant Version"=w90:string[], "main state cluster.Store Data.Inalfa Part Number ECU"=w78:string[], "main state cluster.Store Data.Communication Line 1"=w88:sgl[], "main state cluster.Store Data.Communication Line 2"=w79:sgl[], "main state cluster.Store Data.LVDT Data"=w86:sgl[], "main state cluster.Store Data.Sunshade Close Data"=w72:sgl[], "main state cluster.Store Data.Sun Shade Close Force Limits.Check Noise"=w85:bool, "main state cluster.Store Data.Sunshade Open Data"=w84:sgl[], "main state cluster.Store Data.Sun Shade Open Force Limits.Check Noise"=w83:bool, "main state cluster.Store Data.Anti Pinch Vent Force"=w74:sgl[], "main state cluster.Store Data.iGPS LVDT Data"=w71:sgl[])
        n14 = case shown="假" w63 {
          tunnel: [w125 w128] -> w89
          tunnel: w88 -> [w124 w127]
          tunnel: w86 -> [w123 _]
          tunnel: w79 -> [w122 w126]
          tunnel: w72 -> [w121 _]
          tunnel: w71 -> [w120 _]
          frame True {
            n15 = Build Array (concatenate)(w124, w122, w123, w120, w121) -> (w125:sgl[])
          }
          frame False {
            n16 = Build Array (concatenate)(w127, w126) -> (w128:sgl[])
          }
        }
        n17 = for {
          tunnel: w93 -> [w148] mode=indexing
          tunnel: [w146] -> w92 mode=indexing
          shift-right: [w144] -> w69
          shift-left: w70 -> [w145]
          n18 = Format Into String(format string="%0.3f", error in=w145, w148) -> (resulting string=w146:string, error out=w144:errorcluster)  [unwired: 1 in]
        }
        n19 = for {
          tunnel: w89 -> [w143] mode=indexing
          tunnel: [w141] -> w87 mode=indexing
          shift-right: [w139] -> w68
          shift-left: w69 -> [w140]
          n20 = Format Into String(format string="%0.3f", error in=w140, w143) -> (resulting string=w141:string, error out=w139:errorcluster)  [unwired: 1 in]
        }
        n21 = Format Into String(error in=w68, w85) -> (resulting string=w82:string, error out=w67:errorcluster)  [unwired: 2 in]
        n22 = for {
          tunnel: w84 -> [w138] mode=indexing
          tunnel: [w136] -> w81 mode=indexing
          shift-right: [w134] -> w66
          shift-left: w67 -> [w135]
          n23 = Format Into String(format string="%0.3f", error in=w135, w138) -> (resulting string=w136:string, error out=w134:errorcluster)  [unwired: 1 in]
        }
        n24 = Format Into String(error in=w66, w83) -> (resulting string=w62:string, error out=w65:errorcluster)  [unwired: 2 in]
        n25 = for {
          tunnel: w74 -> [w133] mode=indexing
          tunnel: [w131] -> w73 mode=indexing
          shift-right: [w129] -> w64
          shift-left: w65 -> [w130]
          n26 = Format Into String(format string="%0.3f", error in=w130, w133) -> (resulting string=w131:string, error out=w129:errorcluster)  [unwired: 1 in]
        }
        n27 = Initialize Array("Spare", 7 ("dimension size")) -> (w75:string[])
        n28 = case shown="假" w63 {
          tunnel: w97 -> [w111 w119]
          tunnel: [w110 w118] -> w94
          tunnel: w92 -> [w109 w117]
          tunnel: w91 -> [w108 w116]
          tunnel: w90 -> [w107 w115]
          tunnel: w87 -> [w106 w114]
          tunnel: w82 -> [w105 _]
          tunnel: w81 -> [w104 _]
          tunnel: w62 -> [w103 _]
          tunnel: w80 -> [w102 w113]
          tunnel: w78 -> [w101 w112]
          tunnel: w75 -> [w100 _]
          tunnel: w73 -> [w99 _]
          frame True {
            n29 = Build Array (concatenate)(w102, w109, w111, w108, w107, w101, w106, w105, w104, w103, w99, w100) -> (w110:string[])
          }
          frame False {
            (unwired) ""
            n30 = Build Array (concatenate)(w113, w117, w119, w116, w115, w112, w114) -> (w118:string[])
          }
        }
        n31 = Bundle By Name(cluster=w96, "Excel Data Array"=w94) -> (w95:T35)
      }
      frame "Excel Data 3" {
        n32 = Unbundle By Name(w159) -> ("Excel Data Array"=w156:string[], "main state cluster.Store Data.Motion Data Array"=w155:T11[])
        n33 = for {
          tunnel: w155 -> [w188] mode=indexing
          tunnel: [w170] -> w152 mode=indexing
          tunnel: [w181] -> w151 mode=indexing
          shift-right: [w172] -> w153
          shift-left: string[] [] -> [w171]
          shift-right: [w169] -> w149
          shift-left: w150 -> [w168]
          n34 = Unbundle By Name(w188) -> ("Motion"=w187:T3, "Actual PS Voltage"=w185:dbl, "Switch 1 to 6"=w184:dbl[], "Actual Avg Current"=w183:dbl, "Motion Data Limits.Min Avg Current"=w180:dbl, "Motion Data Limits.Max Avg Current"=w165:dbl, "Actual max Current"=w164:dbl, "Motion Data Limits.Min max Current"=w166:dbl, "Motion Data Limits.Max max Current"=w167:dbl, "Actual Runtime"=w179:dbl, "Motion Data Limits.Max Run Time"=w178:dbl, "Actual Speed"=w177:dbl, "Motion Data Limits.Min Speed"=w176:dbl, "Actual Noise (dB)"=w163:dbl, "Motion Data Limits.Min Sound (dB)"=w162:dbl, "Motion Data Limits.Max Sound (dB)"=w161:dbl, "Motion Data Limits.Check Sound Test"=w182:bool, "AP Data"=w170:i16[][], "Current Data"=w181:sgl[])
          n35 = Build Array (concatenate)(w185, w184, w183, w180, w165, w164, w166, w167, w179, w178, w177, w176, w163, w162, w161) -> (w186:dbl[])
          n36 = for {
            tunnel: w186 -> [w193] mode=indexing
            tunnel: [w191] -> w174 mode=indexing
            shift-right: [w189] -> w169
            shift-left: w168 -> [w190]
            n37 = Format Into String(format string="%0.3f", error in=w190, w193) -> (resulting string=w191:string, error out=w189:errorcluster)  [unwired: 1 in]
          }
          n38 = Format Into String(w187) -> (resulting string=w175:string)  [unwired: 3 in, 1 out]
          n39 = Format Into String(w182) -> (resulting string=w173:string)  [unwired: 3 in, 1 out]
          n40 = Build Array (concatenate)(w171, w175, w174, w173) -> (w172:string[])
        }
        n41 = Build Array (concatenate)(w156, w153) -> (w157:string[])
        n42 = Bundle By Name(cluster=w159, "Excel Data Array"=w157, "AP Data"=w152, "Current Data"=w151) -> (w158:T35)
      }
      frame "Exit" {
      }
      frame "Init" {
        n43 = Unbundle By Name(w239) -> ("main state cluster.misc station config.Station Name"=w202:string, "main state cluster.paths.network path"=w216:path)
        n44 = call "check network path availability.vi"("error in"=w213, "Network Path"=w216) -> ("error out"=w217:errorcluster, "base path"=w215:path)  [unwired: 8 in]
        n45 = Format Date/Time String(time format string (%c)="%Y-%b") -> (date/time string=w235:string)  [unwired: 2 in]
        n46 = Concatenate Strings(w202, "\\Red Rabbit Excel Data\\") -> (w209:string)
        n47 = Build Path(base path=w215, name or relative path=w235) -> (appended path=w200:path)
        n48 = Concatenate Strings(w202, "\\BMW Hall Log\\" ("Audit")) -> (w197:string)
        n49 = Concatenate Strings(w202, "\\Data Bytes Log\\" ("Audit")) -> (w203:string)
        n50 = Concatenate Strings(w202, "\\Excel Data\\" ("Audit")) -> (w229:string)
        n51 = Concatenate Strings(w202, "\\AP Data\\") -> (w228:string)
        n52 = Concatenate Strings(w202, "\\Current Data\\") -> (w227:string)
        n53 = Concatenate Strings(w202, "\\Sunshade Force Data\\") -> (w226:string)
        n54 = Concatenate Strings(w202, "\\Analog Data\\") -> (w210:string)
        n55 = Concatenate Strings(w202, "\\Route To Repair Excel Data\\") -> (w205:string)
        n56 = Build Path(base path=w200, name or relative path=w229) -> (appended path=w204:path)
        n57 = Build Path(base path=w200, name or relative path=w228) -> (appended path=w225:path)
        n58 = Build Path(base path=w200, name or relative path=w227) -> (appended path=w224:path)
        n59 = Build Path(base path=w200, name or relative path=w226) -> (appended path=w223:path)
        n60 = Build Path(base path=w200, name or relative path=w203) -> (appended path=w199:path)
        n61 = Build Path(base path=w200, name or relative path=w210) -> (appended path=w218:path)
        n62 = Build Path(base path=w200, name or relative path=w197) -> (appended path=w198:path)
        n63 = Build Path(base path=w200, name or relative path=w209) -> (appended path=w208:path)
        n64 = Build Path(base path=w200, name or relative path=w205) -> (appended path=w206:path)
        n65 = Build Array(w200, w198, w199, w204, w225, w224, w223, w218, w208, w206) -> (w220:path[])
        n66 = for {
          tunnel: [w244] -> w222 mode=indexing
          tunnel: w220 -> [w241] mode=indexing
          shift-right: [w240] -> w212
          shift-left: w217 -> [w243]
          n67 = call <vilib>:"Check if File or Folder Exists.vi"("error in (no error)"=w243, "path"=w241) -> ("error out"=w242:errorcluster, "file or folder exists?"=w246:bool, "dup path"=w245:path)  [unwired: 7 in]
          n68 = case shown="假" w246 {
            tunnel: w245 -> [w248 w252]
            tunnel: [w248 w251] -> w244
            tunnel: [w247 w250] -> w240
            tunnel: w242 -> [w247 w249]
            frame True {
            }
            frame False {
              n69 = Create Folder(path (use dialog)=w252, error in=w249) -> (created path=w251:path, error out=w250:errorcluster)  [unwired: 1 in, 1 out]
            }
          }
        }
        n70 = call "date and time info.vi"() -> ("Output String"=w214:string)  [unwired: 11 in]
        n71 = Index Array(array=w222) -> (element=w221:path)  [unwired: 1 in]
        n72 = Bundle By Name(cluster=w239, "Date n Time"=w214, "Relative Path Data Bytes Log"=w203, "Relative Path Excel Data"=w229, "Relative Path AP Data"=w228, "Relative Path Current Data"=w227, "Relative Path Sunshade Force Data"=w226, "Base Path"=w221, "Relative Path Analog Data"=w210, "Red Rabbit Relative Path Excel Data"=w209, "Route to repair relative path excel data"=w205, "bmw hall log relative path"=w197) -> (w238:T35)
      }
      frame "Move Data Bytes Log" {
        w262 = "_" ("string")
        n73 = Unbundle By Name(w261) -> ("Base Path"=w277:path, "Relative Path Data Bytes Log"=w276:string, "main state cluster.Store Data.data bytes log"=w256:string)  [unwired: 1 out]
        n74 = Unbundle By Name(w261) -> ("main state cluster.misc status.Part Setup.Part Type"=w260:string, "main state cluster.Store Data.Module Info.Serial Number"=w263:string, "Date n Time"=w265:string)
        n75 = Concatenate Strings(w260, w262, w263, w262, w265, ".txt" ("string")) -> (w259:string)
        n76 = Build Path(base path=w277, name or relative path=w276) -> (appended path=w281:path)
        n77 = call <vilib>:"Check if File or Folder Exists.vi"("error in (no error)"=w266, "path"=w281) -> ("error out"=w279:errorcluster, "file or folder exists?"=w280:bool, "dup path"=w278:path)  [unwired: 7 in]
        n78 = case shown="假" w280 {
          tunnel: w279 -> [w291 w292]
          tunnel: w278 -> [w289 w293]
          tunnel: [w290 w292] -> _
          tunnel: [w288 w293] -> w274
          frame False {
            n79 = Create Folder(path (use dialog)=w289, error in=w291) -> (created path=w288:path, error out=w290:errorcluster)  [unwired: 1 in, 1 out]
          }
          frame True {
          }
        }
        n80 = Format Date/Time String(time format string (%c)="%b %d %Y") -> (date/time string=w268:string)  [unwired: 2 in]
        n81 = Build Path(base path=w274, name or relative path=w268) -> (appended path=w273:path)
        n82 = call <vilib>:"Check if File or Folder Exists.vi"("path"=w273) -> ("error out"=w270:errorcluster, "file or folder exists?"=w272:bool, "dup path"=w271:path)  [unwired: 8 in]
        n83 = case shown="假" w272 {
          tunnel: w270 -> [w285 w286]
          tunnel: w271 -> [w283 w287]
          tunnel: [w284 w286] -> w258
          tunnel: [w282 w287] -> w267
          frame False {
            n84 = Create Folder(path (use dialog)=w283, error in=w285) -> (created path=w282:path, error out=w284:errorcluster)  [unwired: 1 in, 1 out]
          }
          frame True {
          }
        }
        n85 = Build Path(base path=w267, name or relative path=w259) -> (appended path=w257:path)
        n86 = Write to Text File(file (use dialog)=w257, text=w256, error in=w258) -> (refnum out=w254:refnum<file>, error out=w255:errorcluster)  [unwired: 1 in, 1 out]
        n87 = Close File(refnum=w254, error in=w255) -> (error out=w253:errorcluster)  [unwired: 1 out]
      }
      frame "Store Current Data" {
        w301 = "_" ("string")
        # "Temporary directory with data file"
        n88 = Unbundle By Name(w296) -> ("Base Path"=w306:path, "main state cluster.misc status.Part Setup.Part Type"=w304:string, "main state cluster.Store Data.Module Info.Serial Number"=w303:string, "Relative Path Current Data"=w302:string, "Date n Time"=w307:string, "Current Data"=w297:sgl[][])
        n89 = Concatenate Strings(w302, w304, w301, w303, w301, w307, ".zip" ("string")) -> (w299:string)
        n90 = for {
          tunnel: w297 -> [w335] mode=indexing
          tunnel: [w339] -> w318 mode=indexing
          n91 = Array Size(array=w335) -> (size(s)=w341:i32)
          n92 = Reverse 1D Array(array=w335) -> (reversed array=w343:sgl[])
          n93 = while {
            tunnel: w343 -> [w350] mode=indexing
            tunnel: [w348] -> w342
            tunnel: w341 -> [w347]
            i -> [w348]
            stop <- w344 stop-if-true
            n94 = Greater Or Equal?(x=w350, y=sgl 0.5) -> (x >= y?=w345:bool)
            n95 = Greater?(x=w348, y=w347) -> (0:w346:bool)
            n96 = Or(x=w345, y=w346) -> (x .or. y?=w344:bool)
          }
          n97 = Subtract(x=w341, y=w342) -> (x-y=w336:i32)
          n98 = Add(x=w336, y=20 ("x")) -> (x+y=w338:i32)
          n99 = Array Subset(array=w335, index=0, length=w338) -> (w339:sgl[])
        }
        n100 = Build Path(base path=w306, name or relative path=w299) -> (appended path=w300:path)
        n101 = call "Check R Create Dir.vi"("File Path"=w300) -> ("Dir Path"=w298:path)  [unwired: 10 in]
        n102 = call <vilib>:"Get File Extension.vi"("file"=w298) -> ("filename without extension"=w309:string)  [unwired: 6 in, 4 out]
        n103 = call <vilib>:"New Zip File.vi"("error in (no error)"=w294, "target"=w298) -> ("error out"=w329:errorcluster, "zip file out"=w328:i64)  [unwired: 3 in, 1 out]
        n104 = String Subset(string=w309, offset (0)=2) -> (substring=w308:string)  [unwired: 1 in]
        n105 = Temporary Directory() -> (w315:path)
        n106 = Build Path(base path=w315, name or relative path=w308) -> (appended path=w316:path)
        n107 = Flatten To String(anything=w318) -> (data string=w334:string)  [unwired: 3 in, 2 out]
        n108 = Write to Text File(file (use dialog)=w316, text=w334) -> (refnum out=w311:refnum<file>)  [unwired: 2 in, 2 out]
        n109 = Refnum to Path(1:w311) -> (0:w317:path)
        n110 = Strip Path(path=w317) -> (stripped path=w324:path)  [unwired: 1 out]
        n111 = Path to Array of Strings(0:w324) -> (2:w323:string[])  [unwired: 1 out]
        n112 = Path to Array of Strings(0:w317) -> (2:w325:string[])  [unwired: 1 out]
        n113 = Array Size(array=w323) -> (size(s)=w322:i32)
        n114 = call "Insert Multiple Events.vi"("Insert all? (T)"="Store Sunshade Raw Data?", "Events to Insert"=string[] ["Store Sunshade Raw Data"], "Event queue in"=w333) -> ("Event queue out"=w332:string[])  [unwired: 4 in]
        n115 = Array Subset(array=w325, index=w322) -> (w321:string[])  [unwired: 1 in]
        n116 = Array of Strings to Path(0:w321, 1:TRUE ("relative")) -> (2:w320:path)
        n117 = call <vilib>:"Add File to Zip.vi"("error in (no error)"=w329, "destination path in zip"=w320, "source file path"=w317, "zip file in"=w328) -> ("error out"=w327:errorcluster, "zip file out"=w326:i64)  [unwired: 6 in]
        n118 = call <vilib>:"Close Zip File.vi"("error in (no error)"=w327, "zip file in"=w326) -> ("error out"=w313:errorcluster)  [unwired: 5 in]
        n119 = Close File(refnum=w311, error in=w313) -> (path=w314:path, error out=w312:errorcluster)
        n120 = Delete(path (use dialog)=w314, error in=w312) -> (error out=w295:errorcluster)  [unwired: 3 in, 2 out]
      }
      frame "Store Data Into Files" {
        w373 = "_" ("string")
        # "Every day new directory is created"
        # "From temporary file pat, get filename without extention"
        n121 = Unbundle By Name(w354) -> ("Red Rabbit Relative Path Excel Data"=w362:string, "main state cluster.Sequence State.Red-Rabbit Mode"=w363:bool, "Route to repair relative path excel data"=w359:string, "main state cluster.Sequence State.route-to-repair mode"=w361:bool, "Relative Path Excel Data"=w360:string, "Excel Data Array"=w353:string[], "AP Data"=w402:i16[][][])  [unwired: 1 out]
        n122 = Unbundle By Name(w354) -> ("Base Path"=w356:path, "Relative Path AP Data"=w366:string, "main state cluster.misc status.Part Setup.Part Type"=w369:string, "main state cluster.Store Data.Module Info.Serial Number"=w370:string, "Date n Time"=w367:string)
        n123 = Temporary Directory() -> (w382:path)
        n124 = Select(t=w359, s=w361, f=w360) -> (s? t:f=w358:string)
        n125 = Flatten To String(anything=w402) -> (data string=w403:string)  [unwired: 3 in, 2 out]
        n126 = Select(t=w362, s=w363, f=w358) -> (s? t:f=w357:string)
        n127 = Concatenate Strings(w366, w369, w373, w370, w373, w367, ".zip" ("string")) -> (w371:string)
        n128 = case shown="假" w351 {
          tunnel: [string[] ["Serial Number", "Pallet Number", "Date and Time", "Part Type", "Pass/Fail", "Error Table", "Sunsahde Color", "Station Name", "Run Time", "AP Cycle PS Voltage", "AP Force Glass", "AP Force Glass Lt", "AP Force Sunshade", "AP Force Sunshade Lt", "AP Force Sunshade02", "AP Force Sunshade02 Lt", "AP Force Glass Vent ", "AP Force Glass Vent Lt", "SW Version", "SW Version Lt", "HW Version", "HW Version Lt", "Constant Version", "Constant Version Lt", "Inalfa Part Number", "Inalfa Part Number Lt", "Commu Line 1", "Commu Line 1 Lt", "Delta Commu Line 1", "Commu Line 2", "Commu Line 2 Lt", "Delta Commu Line 2", "LVDT 1", "LVDT 1 Min Lt", "LVDT 1 Max Lt", "LVDT 2", "LVDT 2 Min Lt", "LVDT 2 Max Lt", "LVDT 3", "LVDT 3 Min Lt", "LVDT 3 Max Lt", "LVDT 4", "LVDT 4 Min Lt", "LVDT 4 Max Lt", "LVDT 5", "LVDT 5 Min Lt", "LVDT 5 Max Lt", "LVDT 6", "LVDT 6 Min Lt", "LVDT 6 Max Lt", "LVDT 7", "LVDT 7 Min Lt", "LVDT 7 Max Lt", "LVDT 8", "LVDT 8 Min Lt", "LVDT 8 Max Lt", "LVDT 9", "LVDT 9 Min Lt", "LVDT 9 Max Lt", "LVDT 10", "LVDT 10 Min Lt", "LVDT 10 Max Lt", "LVDT 11", "LVDT 11 Min Lt", "LVDT 11 Max Lt", "LVDT 12", "LVDT 12 Min Lt", "LVDT 12 Max Lt", "LVDT 13", "LVDT 13 Min Lt", "LVDT 13 Max Lt", "LVDT 14", "LVDT 14 Min Lt", "LVDT 14 Max Lt", "LVDT 15", "LVDT 15 Min Lt", "LVDT 15 Max Lt", "iGPS LVDT 1", "iGPS LVDT 1 Min Lt", "iGPS LVDT 1 Max Lt", "iGPS LVDT 2", "iGPS LVDT 2 Min Lt", "iGPS LVDT 2 Max Lt", "iGPS LVDT 3", "iGPS LVDT 3 Min Lt", "iGPS LVDT 3 Max Lt", "iGPS LVDT 4", "iGPS LVDT 4 Min Lt", "iGPS LVDT 4 Max Lt", "iGPS LVDT 5", "iGPS LVDT 5 Min Lt", "iGPS LVDT 5 Max Lt", "iGPS LVDT 6", "iGPS LVDT 6 Min Lt", "iGPS LVDT 6 Max Lt", "iGPS LVDT 7", "iGPS LVDT 7 Min Lt", "iGPS LVDT 7 Max Lt", "iGPS LVDT 8", "iGPS LVDT 8 Min Lt", "iGPS LVDT 8 Max Lt", "iGPS LVDT 9", "iGPS LVDT 9 Min Lt", "iGPS LVDT 9 Max Lt", "iGPS LVDT 10", "iGPS LVDT 10 Min Lt", "iGPS LVDT 10 Max Lt", "iGPS LVDT 11", "iGPS LVDT 11 Min Lt", "iGPS LVDT 11 Max Lt", "iGPS LVDT 12", "iGPS LVDT 12 Min Lt", "iGPS LVDT 12 Max Lt", "iGPS LVDT 13", "iGPS LVDT 13 Min Lt", "iGPS LVDT 13 Max Lt", "iGPS LVDT 14", "iGPS LVDT 14 Min Lt", "iGPS LVDT 14 Max Lt", "iGPS LVDT 15", "iGPS LVDT 15 Min Lt", "iGPS LVDT 15 Max Lt", "SH Close Min", "SH Close Min Lt", "SH Close Max", "SH Close Max Lt", "SH Close Avg Min", "SH Close Avg Min Lt", "SH Close Avg Max", "SH Close Avg Max Lt", "SH Close Variance", "SH Close Variance Lt", "SH Close Noise Check?", "SH Open Min", "SH Open Min Lt", "SH Open Max", "SH Open Max Lt", "SH Open Avg Min", "SH Open Avg Min Lt", "SH Open Avg Max", "SH Open Avg Max Lt", "SH Open Variance", "SH Open Variance Lt", "SH Open Noise Check?", "AP Vent Force", "AP Vent Force Min Lt", "AP Vent Force Max Lt", "Spare Field 1", "Spare Field 2", "Spare Field 3", "Spare Field 4", "Spare Field 5", "Spare Field 6", "Spare Field 7", "Motion", "PS Voltage", "Switch 1", "Switch 2", "Switch 3", "Switch 4", "Switch 5", "Switch 6", "Switch 7", "Switch 8", "Avg Current", "Avg Current Min Lt", "Avg Current Max Lt", "Max Current", "Max Current Min Lt", "Max Current Max Lt", "Run Time", "Run Time Max", "Speed", "Speed Min Lt", "Device Noise (dB)", "Device Noise Min Lt ", "Device Noise Max Lt ", "Noise Test Tested?", "Motion", "PS Voltage", "Switch 1", "Switch 2", "Switch 3", "Switch 4", "Switch 5", "Switch 6", "Switch 7", "Switch 8", "Avg Current", "Avg Current Min Lt", "Avg Current Max Lt", "Max Current", "Max Current Min Lt", "Max Current Max Lt", "Run Time", "Run Time Max", "Speed", "Speed Min Lt", "Device Noise (dB)", "Device Noise Min Lt ", "Device Noise Max Lt ", "Noise Test Tested?", "Motion", "PS Voltage", "Switch 1", "Switch 2", "Switch 3", "Switch 4", "Switch 5", "Switch 6", "Switch 7", "Switch 8", "Avg Current", "Avg Current Min Lt", "Avg Current Max Lt", "Max Current", "Max Current Min Lt", "Max Current Max Lt", "Run Time", "Run Time Max", "Speed", "Speed Min Lt", "Device Noise (dB)", "Device Noise Min Lt ", "Device Noise Max Lt ", "Noise Test Tested?", "Motion", "PS Voltage", "Switch 1", "Switch 2", "Switch 3", "Switch 4", "Switch 5", "Switch 6", "Switch 7", "Switch 8", "Avg Current", "Avg Current Min Lt", "Avg Current Max Lt", "Max Current", "Max Current Min Lt", "Max Current Max Lt", "Run Time", "Run Time Max", "Speed", "Speed Min Lt", "Device Noise (dB)", "Device Noise Min Lt ", "Device Noise Max Lt ", "Noise Test Tested?", "Motion", "PS Voltage", "Switch 1", "Switch 2", "Switch 3", "Switch 4", "Switch 5", "Switch 6", "Switch 7", "Switch 8", "Avg Current", "Avg Current Min Lt", "Avg Current Max Lt", "Max Current", "Max Current Min Lt", "Max Current Max Lt", "Run Time", "Run Time Max", "Speed", "Speed Min Lt", "Device Noise (dB)", "Device Noise Min Lt ", "Device Noise Max Lt ", "Noise Test Tested?", "Motion", "PS Voltage", "Switch 1", "Switch 2", "Switch 3", "Switch 4", "Switch 5", "Switch 6", "Switch 7", "Switch 8", "Avg Current", "Avg Current Min Lt", "Avg Current Max Lt", "Max Current", "Max Current Min Lt", "Max Current Max Lt", "Run Time", "Run Time Max", "Speed", "Speed Min Lt", "Device Noise (dB)", "Device Noise Min Lt ", "Device Noise Max Lt ", "Noise Test Tested?", "Motion", "PS Voltage", "Switch 1", "Switch 2", "Switch 3", "Switch 4", "Switch 5", "Switch 6", "Switch 7", "Switch 8", "Avg Current", "Avg Current Min Lt", "Avg Current Max Lt", "Max Current", "Max Current Min Lt", "Max Current Max Lt", "Run Time", "Run Time Max", "Speed", "Speed Min Lt", "Device Noise (dB)", "Device Noise Min Lt ", "Device Noise Max Lt ", "Noise Test Tested?", "Motion", "PS Voltage", "Switch 1", "Switch 2", "Switch 3", "Switch 4", "Switch 5", "Switch 6", "Switch 7", "Switch 8", "Avg Current", "Avg Current Min Lt", "Avg Current Max Lt", "Max Current", "Max Current Min Lt", "Max Current Max Lt", "Run Time", "Run Time Max", "Speed", "Speed Min Lt", "Device Noise (dB)", "Device Noise Min Lt ", "Device Noise Max Lt ", "Noise Test Tested?", "Motion", "PS Voltage", "Switch 1", "Switch 2", "Switch 3", "Switch 4", "Switch 5", "Switch 6", "Switch 7", "Switch 8", "Avg Current", "Avg Current Min Lt", "Avg Current Max Lt", "Max Current", "Max Current Min Lt", "Max Current Max Lt", "Run Time", "Run Time Max", "Speed", "Speed Min Lt", "Device Noise (dB)", "Device Noise Min Lt ", "Device Noise Max Lt ", "Noise Test Tested?", "Motion", "PS Voltage", "Switch 1", "Switch 2", "Switch 3", "Switch 4", "Switch 5", "Switch 6", "Switch 7", "Switch 8", "Avg Current", "Avg Current Min Lt", "Avg Current Max Lt", "Max Current", "Max Current Min Lt", "Max Current Max Lt", "Run Time", "Run Time Max", "Speed", "Speed Min Lt", "Device Noise (dB)", "Device Noise Min Lt ", "Device Noise Max Lt ", "Noise Test Tested?"] ("output array") string[] ["Serial Number", "Pallet Number", "Date and Time", "Part Type", "Pass/Fail", "Error Table", "Sunsahde Color", "Station Name", "Run Time", "AP Cycle PS Voltage", "AP Force Glass", "AP Force Glass Lt", "AP Force Sunshade", "AP Force Sunshade Lt", "AP Force Sunshade02", "AP Force Sunshade02 Lt", "AP Force Glass Vent ", "AP Force Glass Vent Lt", "SW Version", "SW Version Lt", "HW Version", "HW Version Lt", "Constant Version", "Constant Version Lt", "Inalfa Part Number", "Inalfa Part Number Lt", "Commu Line 1", "Commu Line 1 Lt", "Delta Commu Line 1", "Commu Line 2", "Commu Line 2 Lt", "Delta Commu Line 2", "Motion", "PS Voltage", "Switch 1", "Switch 2", "Switch 3", "Switch 4", "Switch 5", "Switch 6", "Switch 7", "Switch 8", "Avg Current", "Avg Current Min Lt", "Avg Current Max Lt", "Max Current", "Max Current Min Lt", "Max Current Max Lt", "Run Time", "Run Time Max", "Speed", "Speed Min Lt", "Device Noise (dB)", "Device Noise Min Lt ", "Device Noise Max Lt ", "Noise Test Tested?", "Motion", "PS Voltage", "Switch 1", "Switch 2", "Switch 3", "Switch 4", "Switch 5", "Switch 6", "Switch 7", "Switch 8", "Avg Current", "Avg Current Min Lt", "Avg Current Max Lt", "Max Current", "Max Current Min Lt", "Max Current Max Lt", "Run Time", "Run Time Max", "Speed", "Speed Min Lt", "Device Noise (dB)", "Device Noise Min Lt ", "Device Noise Max Lt ", "Noise Test Tested?", "Motion", "PS Voltage", "Switch 1", "Switch 2", "Switch 3", "Switch 4", "Switch 5", "Switch 6", "Switch 7", "Switch 8", "Avg Current", "Avg Current Min Lt", "Avg Current Max Lt", "Max Current", "Max Current Min Lt", "Max Current Max Lt", "Run Time", "Run Time Max", "Speed", "Speed Min Lt", "Device Noise (dB)", "Device Noise Min Lt ", "Device Noise Max Lt ", "Noise Test Tested?", "Motion", "PS Voltage", "Switch 1", "Switch 2", "Switch 3", "Switch 4", "Switch 5", "Switch 6", "Switch 7", "Switch 8", "Avg Current", "Avg Current Min Lt", "Avg Current Max Lt", "Max Current", "Max Current Min Lt", "Max Current Max Lt", "Run Time", "Run Time Max", "Speed", "Speed Min Lt", "Device Noise (dB)", "Device Noise Min Lt ", "Device Noise Max Lt ", "Noise Test Tested?", "Motion", "PS Voltage", "Switch 1", "Switch 2", "Switch 3", "Switch 4", "Switch 5", "Switch 6", "Switch 7", "Switch 8", "Avg Current", "Avg Current Min Lt", "Avg Current Max Lt", "Max Current", "Max Current Min Lt", "Max Current Max Lt", "Run Time", "Run Time Max", "Speed", "Speed Min Lt", "Device Noise (dB)", "Device Noise Min Lt ", "Device Noise Max Lt ", "Noise Test Tested?", "Motion", "PS Voltage", "Switch 1", "Switch 2", "Switch 3", "Switch 4", "Switch 5", "Switch 6", "Switch 7", "Switch 8", "Avg Current", "Avg Current Min Lt", "Avg Current Max Lt", "Max Current", "Max Current Min Lt", "Max Current Max Lt", "Run Time", "Run Time Max", "Speed", "Speed Min Lt", "Device Noise (dB)", "Device Noise Min Lt ", "Device Noise Max Lt ", "Noise Test Tested?", "Motion", "PS Voltage", "Switch 1", "Switch 2", "Switch 3", "Switch 4", "Switch 5", "Switch 6", "Switch 7", "Switch 8", "Avg Current", "Avg Current Min Lt", "Avg Current Max Lt", "Max Current", "Max Current Min Lt", "Max Current Max Lt", "Run Time", "Run Time Max", "Speed", "Speed Min Lt", "Device Noise (dB)", "Device Noise Min Lt ", "Device Noise Max Lt ", "Noise Test Tested?", "Motion", "PS Voltage", "Switch 1", "Switch 2", "Switch 3", "Switch 4", "Switch 5", "Switch 6", "Switch 7", "Switch 8", "Avg Current", "Avg Current Min Lt", "Avg Current Max Lt", "Max Current", "Max Current Min Lt", "Max Current Max Lt", "Run Time", "Run Time Max", "Speed", "Speed Min Lt", "Device Noise (dB)", "Device Noise Min Lt ", "Device Noise Max Lt ", "Noise Test Tested?", "Motion", "PS Voltage", "Switch 1", "Switch 2", "Switch 3", "Switch 4", "Switch 5", "Switch 6", "Switch 7", "Switch 8", "Avg Current", "Avg Current Min Lt", "Avg Current Max Lt", "Max Current", "Max Current Min Lt", "Max Current Max Lt", "Run Time", "Run Time Max", "Speed", "Speed Min Lt", "Device Noise (dB)", "Device Noise Min Lt ", "Device Noise Max Lt ", "Noise Test Tested?", "Motion", "PS Voltage", "Switch 1", "Switch 2", "Switch 3", "Switch 4", "Switch 5", "Switch 6", "Switch 7", "Switch 8", "Avg Current", "Avg Current Min Lt", "Avg Current Max Lt", "Max Current", "Max Current Min Lt", "Max Current Max Lt", "Run Time", "Run Time Max", "Speed", "Speed Min Lt", "Device Noise (dB)", "Device Noise Min Lt ", "Device Noise Max Lt ", "Noise Test Tested?"] ("array w/ subset deleted")] -> w355
          frame True {
          }
          frame False {
          }
        }
        n129 = Build Path(base path=w356, name or relative path=w371) -> (appended path=w372:path)
        n130 = call "Check R Create Dir.vi"("File Path"=w372) -> ("Dir Path"=w365:path)  [unwired: 10 in]
        n131 = call <vilib>:"Get File Extension.vi"("file"=w365) -> ("filename without extension"=w388:string)  [unwired: 6 in, 4 out]
        n132 = Build Path(base path=w382, name or relative path=w388) -> (appended path=w389:path)
        n133 = call <vilib>:"New Zip File.vi"("error in (no error)"=w364, "target"=w365) -> ("error out"=w401:errorcluster, "zip file out"=w400:i64)  [unwired: 3 in, 1 out]
        n134 = Write to Text File(file (use dialog)=w389, text=w403) -> (refnum out=w386:refnum<file>)  [unwired: 2 in, 2 out]
        n135 = Refnum to Path(1:w386) -> (0:w387:path)
        n136 = Strip Path(path=w387) -> (stripped path=w396:path)  [unwired: 1 out]
        n137 = Path to Array of Strings(0:w387) -> (2:w397:string[])  [unwired: 1 out]
        n138 = Path to Array of Strings(0:w396) -> (2:w395:string[])  [unwired: 1 out]
        n139 = Format Date/Time String(time format string (%c)="%b-%d-%y") -> (date/time string=w380:string)  [unwired: 2 in]
        n140 = Array Size(array=w395) -> (size(s)=w394:i32)
        n141 = Concatenate Strings(w357, w380, ".xls" ("string")) -> (w375:string)
        n142 = Array Subset(array=w397, index=w394) -> (w393:string[])  [unwired: 1 in]
        n143 = Array of Strings to Path(0:w393, 1:TRUE ("relative")) -> (2:w392:path)
        n144 = Build Path(base path=w356, name or relative path=w375) -> (appended path=w378:path)
        n145 = call <vilib>:"Add File to Zip.vi"("error in (no error)"=w401, "destination path in zip"=w392, "source file path"=w387, "zip file in"=w400) -> ("error out"=w399:errorcluster, "zip file out"=w398:i64)  [unwired: 6 in]
        n146 = call <vilib>:"Check if File or Folder Exists.vi"("path"=w378) -> ("file or folder exists?"=w377:bool, "dup path"=w376:path)  [unwired: 8 in, 1 out]
        n147 = call <vilib>:"Close Zip File.vi"("error in (no error)"=w399, "zip file in"=w398) -> ("error out"=w385:errorcluster)  [unwired: 5 in]
        n148 = case shown="假" w377 {
          tunnel: w376 -> [w410 w411]
          tunnel: [w409 w411] -> w374
          tunnel: w355 -> [w408 _]
          frame False {
            n149 = call-poly <vilib>:"Write To Spreadsheet File.vi"("append to file? (new file:F)"=FALSE, "1D data"=w408, "file path (dialog if empty)"=w410) -> ("new file path (Not A Path if cancelled)"=w409:path)  [unwired: 5 in]
          }
          frame True {
          }
        }
        n150 = Close File(refnum=w386, error in=w385) -> (path=w383:path, error out=w384:errorcluster)
        n151 = Delete(path (use dialog)=w383, error in=w384) -> (error out=w352:errorcluster)  [unwired: 3 in, 2 out]
        n152 = call-poly <vilib>:"Write To Spreadsheet File.vi"("append to file? (new file:F)"=TRUE, "1D data"=w353, "file path (dialog if empty)"=w374) -> ()  [unwired: 5 in, 1 out]
      }
      frame "Store Sunshade Raw Data" {
        w436 = "_" ("string")
        # "Every day new directory is created"
        n153 = Unbundle By Name(w413) -> ("Base Path"=w432:path, "Relative Path Sunshade Force Data"=w431:string, "main state cluster.misc status.Part Setup.Part Type"=w417:string, "main state cluster.Store Data.Module Info.Serial Number"=w430:string, "Date n Time"=w429:string, "main state cluster.Store Data.Sunsahde Close Raw Data"=w420:sgl[], "main state cluster.Store Data.Sunshade Open Raw Data"=w419:sgl[])
        n154 = Build Array (concatenate)(w420, w419) -> (w416:sgl[])
        n155 = Array Size(array=w416) -> (size(s)=w426:i32)
        n156 = Reverse 1D Array(array=w416) -> (reversed array=w428:sgl[])
        n157 = while {
          tunnel: w428 -> [w444] mode=indexing
          tunnel: [w442] -> w427
          tunnel: w426 -> [w441]
          i -> [w442]
          stop <- w438 stop-if-true
          n158 = Greater Or Equal?(x=w444, y=1.0) -> (x >= y?=w439:bool)
          n159 = Greater?(x=w442, y=w441) -> (0:w440:bool)
          n160 = Or(x=w439, y=w440) -> (x .or. y?=w438:bool)
        }
        n161 = Concatenate Strings(w431, w417, w436, w430, w436, w429) -> (w435:string)
        n162 = Build Path(base path=w432, name or relative path=w435) -> (appended path=w434:path)
        n163 = Subtract(x=w426, y=w427) -> (x-y=w422:i32)
        n164 = Add(x=w422, y=20 ("x")) -> (x+y=w424:i32)
        n165 = call "Check R Create Dir.vi"("File Path"=w434) -> ("Dir Path"=w433:path)  [unwired: 10 in]
        n166 = Array Subset(array=w416, index=0, length=w424) -> (w412:sgl[])
        n167 = Flatten To String(anything=w412, error in (no error)=w415) -> (data string=w421:string, error out=w418:errorcluster)  [unwired: 2 in, 1 out]
        n168 = Write to Text File(file (use dialog)=w433, text=w421, error in=w418) -> (error out=w414:errorcluster)  [unwired: 1 in, 2 out]
      }
      frame "Store Analog Dump" {
        # "for a failed test, store all analog data from the last 60 seconds in addition to the analog data from the last executed motion"
        n169 = Unbundle By Name(w454) -> ("main state cluster.Station Index"=w456:i32, "Relative Path Analog Data"=w446:string, "main state cluster"=w455:T1, "Base Path"=w447:path, "Date n Time"=w445:string)
        n170 = call "dump analog buffer.vi"("Relative Path Current Data"=w446, "Date n Time"=w445, "Base Path"=w447, "error in"=w452, "station idx"=w456, "ain buffer instead of motion buffer"=TRUE, "main state cluster"=w455) -> ("error out"=w448:errorcluster)  [unwired: 4 in]
        n171 = call "dump analog buffer.vi"("Relative Path Current Data"=w446, "Date n Time"=w445, "Base Path"=w447, "error in"=w448, "station idx"=w456, "ain buffer instead of motion buffer"=FALSE, "main state cluster"=w455) -> ("error out"=w451:errorcluster)  [unwired: 4 in]
      }
    }
  }
  "error out" <- w5
